vi "ExGraph.vi"() -> ()   [LabVIEW 2018]
uses:
  Lib/STM/Graph/MOKO_Graph_main_STM.ctl
  Lib/STM/Graph/MOKO_Graph_main_ITEM.ctl
  Lib/STM/Grafic/MOKO_Grafic_STM.ctl
  Lib/STM/Grafic/MOKO_Grafic_ITEM.ctl
  Lib/CTL/STM GRAPH.ctl
  Lib/CTL/Graph settings.ctl
  Lib/CTL/Line.ctl
  <vilib>/Utility/miscctls.llb/LVComboBoxStrsAndValuesArrayTypeDef.ctl
  Lib/Windows/Settings/GraphSettings/GraphSettings_STM.ctl
  Lib/Windows/Settings/GraphSettings/GraphSettings_ITEM.ctl
panel:
  in  "Delete":bool
  in  "Screenshot Indicator":bool
  in  "params":string
  in  "STM Graph":T1={"Graph settings"={"Axis X Min"=0.0, "Axis X Name"="", "Axis X Max"=0.0, "Axis Y Min"=0.0, " Axis Y Name"="", "Axis Y Max"=1.0, "Autoscale"=enum."Yes", "Choice Line"=1.0}, "Lines"=[], "Data"=""} {"Lines"."Color" format="%x"}
  out "MOKO_GRAPH_STM":refnum<queue>
  in  "Combo Box":string(combo)
  in  "Base64 String":string
  out "XY Graph":cluster{"Array Ox":dbl[], "Array Oy":dbl[]}[](graph)
  out "String Array Out":string[](array[string])
  in  "NumPlot":dbl
  out "Counter":dbl
  out "Hide/Show Array":dbl[](array[numeric])
  in  "Config":bool
  in  "Start":bool
  out "MOKO_GRAPH_SERVER":refnum<queue>
  in  "Stop":bool
  out "Boolean":bool
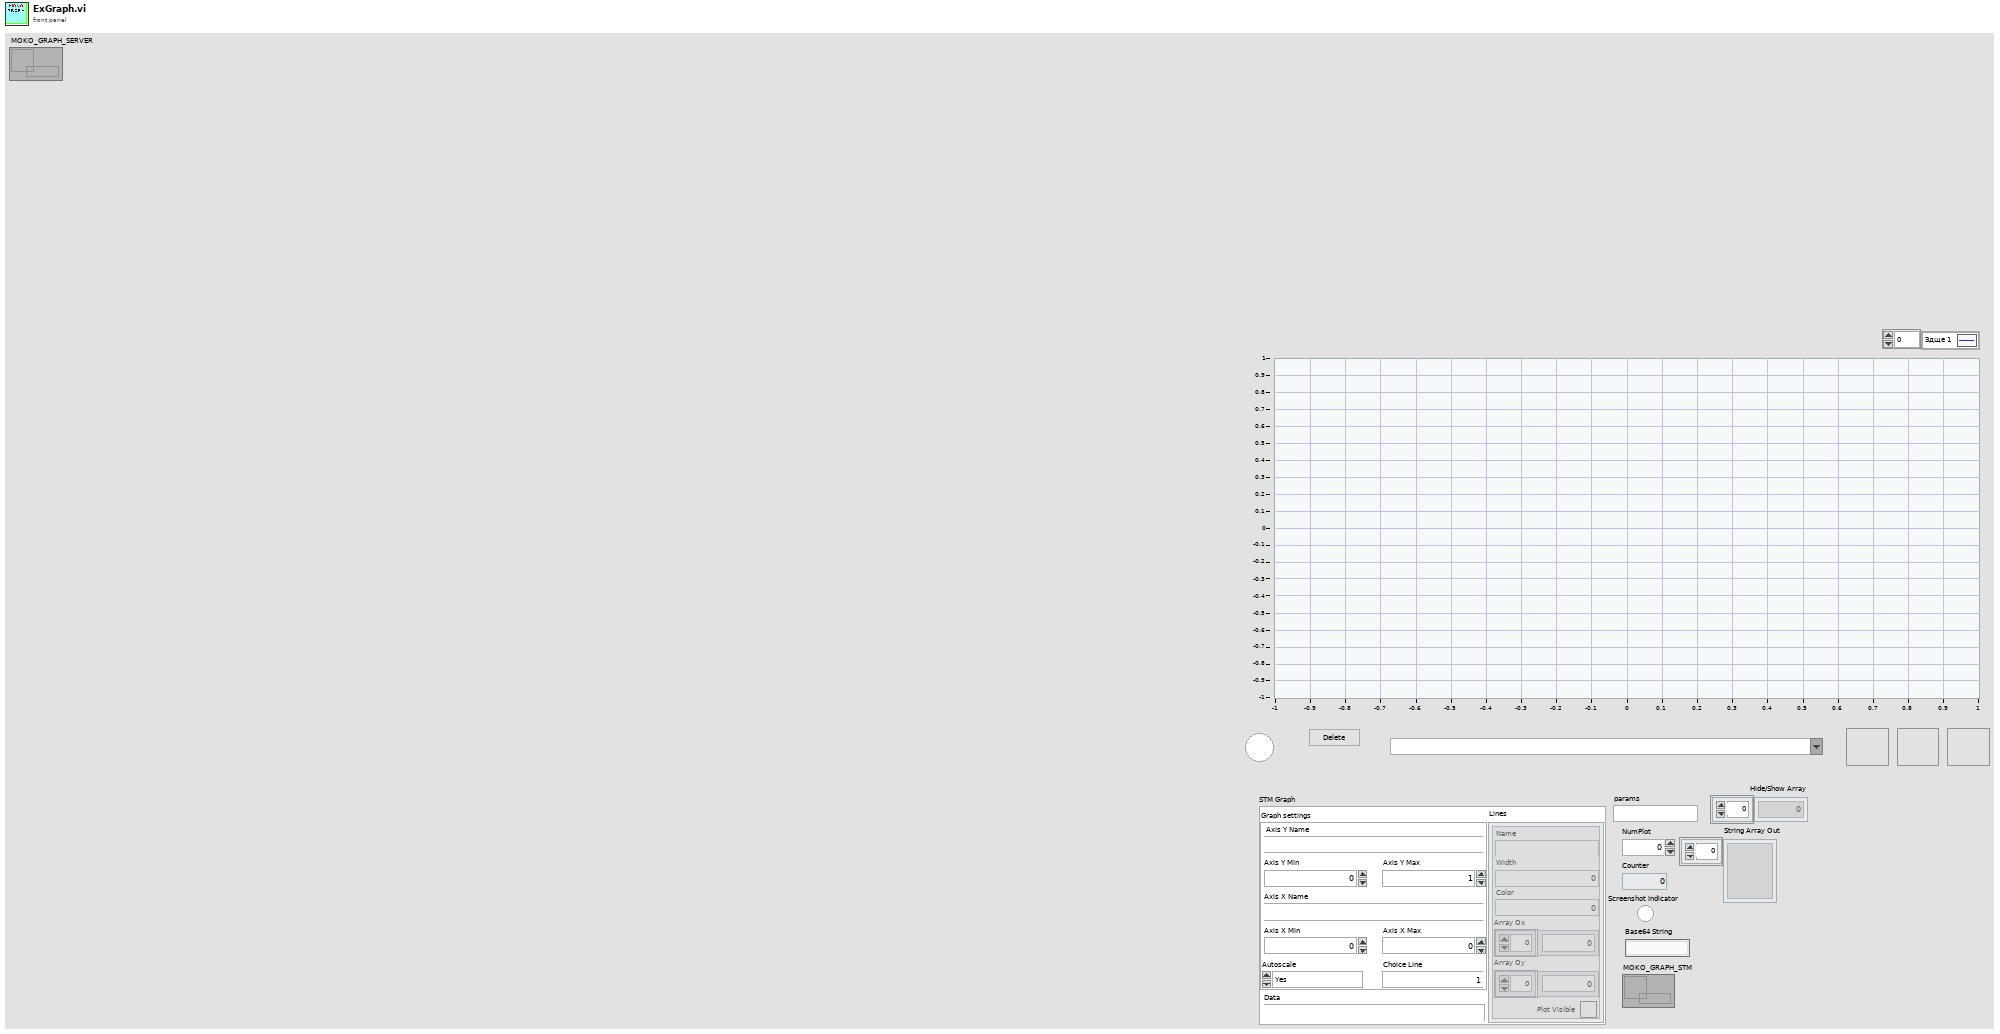
[diagram p1: front panel]
types:
  T1 = typedef "STM GRAPH.ctl" = cluster{"Graph settings":T2, "Lines":T3[], "Data":string}
  T2 = typedef "Graph settings.ctl" = cluster{"Axis X Min":dbl, "Axis X Name":string, "Axis X Max":dbl, "Axis Y Min":dbl, " Axis Y Name":string, "Axis Y Max":dbl, "Autoscale":enum16{"Yes", "No", "Only Oy", "Only Ox"}, "Choice Line":dbl}
  T3 = typedef "Line.ctl" = cluster{"Width":dbl, "Color":i64, "Array Oy":dbl[], "Array Ox":dbl[], "Name":string, "Plot Visible":bool}
  T4 = typedef "MOKO_Grafic_STM.ctl" = cluster{"main stm":T5, "STM Graph":T1}
  T5 = typedef "MOKO_Grafic_ITEM.ctl" = enum16{"idle", "init", "_____ GRAPH STATE_____ ", "Write Graph", "Clear Graph", "close", "Screenshot", "Change Line", "Add Line", "Parse String In", "Add Data", "Change Data", "Graph Settings", "Get Graph Appearance", "Set Graph Appearance", "Delete Data", "Delete Line", "Choose ActPlot", "Set Line Settings", "Increment Smth", "ReWrite Graph", "Autoscale", "Set Autoscale", "Hide Line", "Get Hide Line", "Hide Data", "Show Line", "Get Show Line", "Show Data", "Choose Line", "Change Combo Box", "Send Data", "Receive Data", "Choice Line", "Change Lines"}
  T6 = typedef "MOKO_Graph_main_STM.ctl" = cluster{"main stm":T7, "data":string}
  T7 = typedef "MOKO_Graph_main_ITEM.ctl" = enum16{"idle", "Graph read", "Graph write"}
  T8 = typedef "LVComboBoxStrsAndValuesArrayTypeDef.ctl" = cluster{"String":string, "Value":string}[]
  T9 = typedef "GraphSettings_STM.ctl" = cluster{"main stm":T10, "STM Graph":T1}
  T10 = typedef "GraphSettings_ITEM.ctl" = enum16{"idle", "init", "close", "_____ GRAPH STATE_____ ", "Receive Data", "Send Data", "Change Line", "Delete Line", "Add Line", "Find Max", "Change Color", "Choice Line"}
  T11 = typedef "imagedata.ctl" = cluster{"image type":i32, "image depth":i32, "image":u8[], "mask":u8[], "colors":u32[], "Rectangle":cluster{"left":i16, "top":i16, "right":i16, "bottom":i16}}
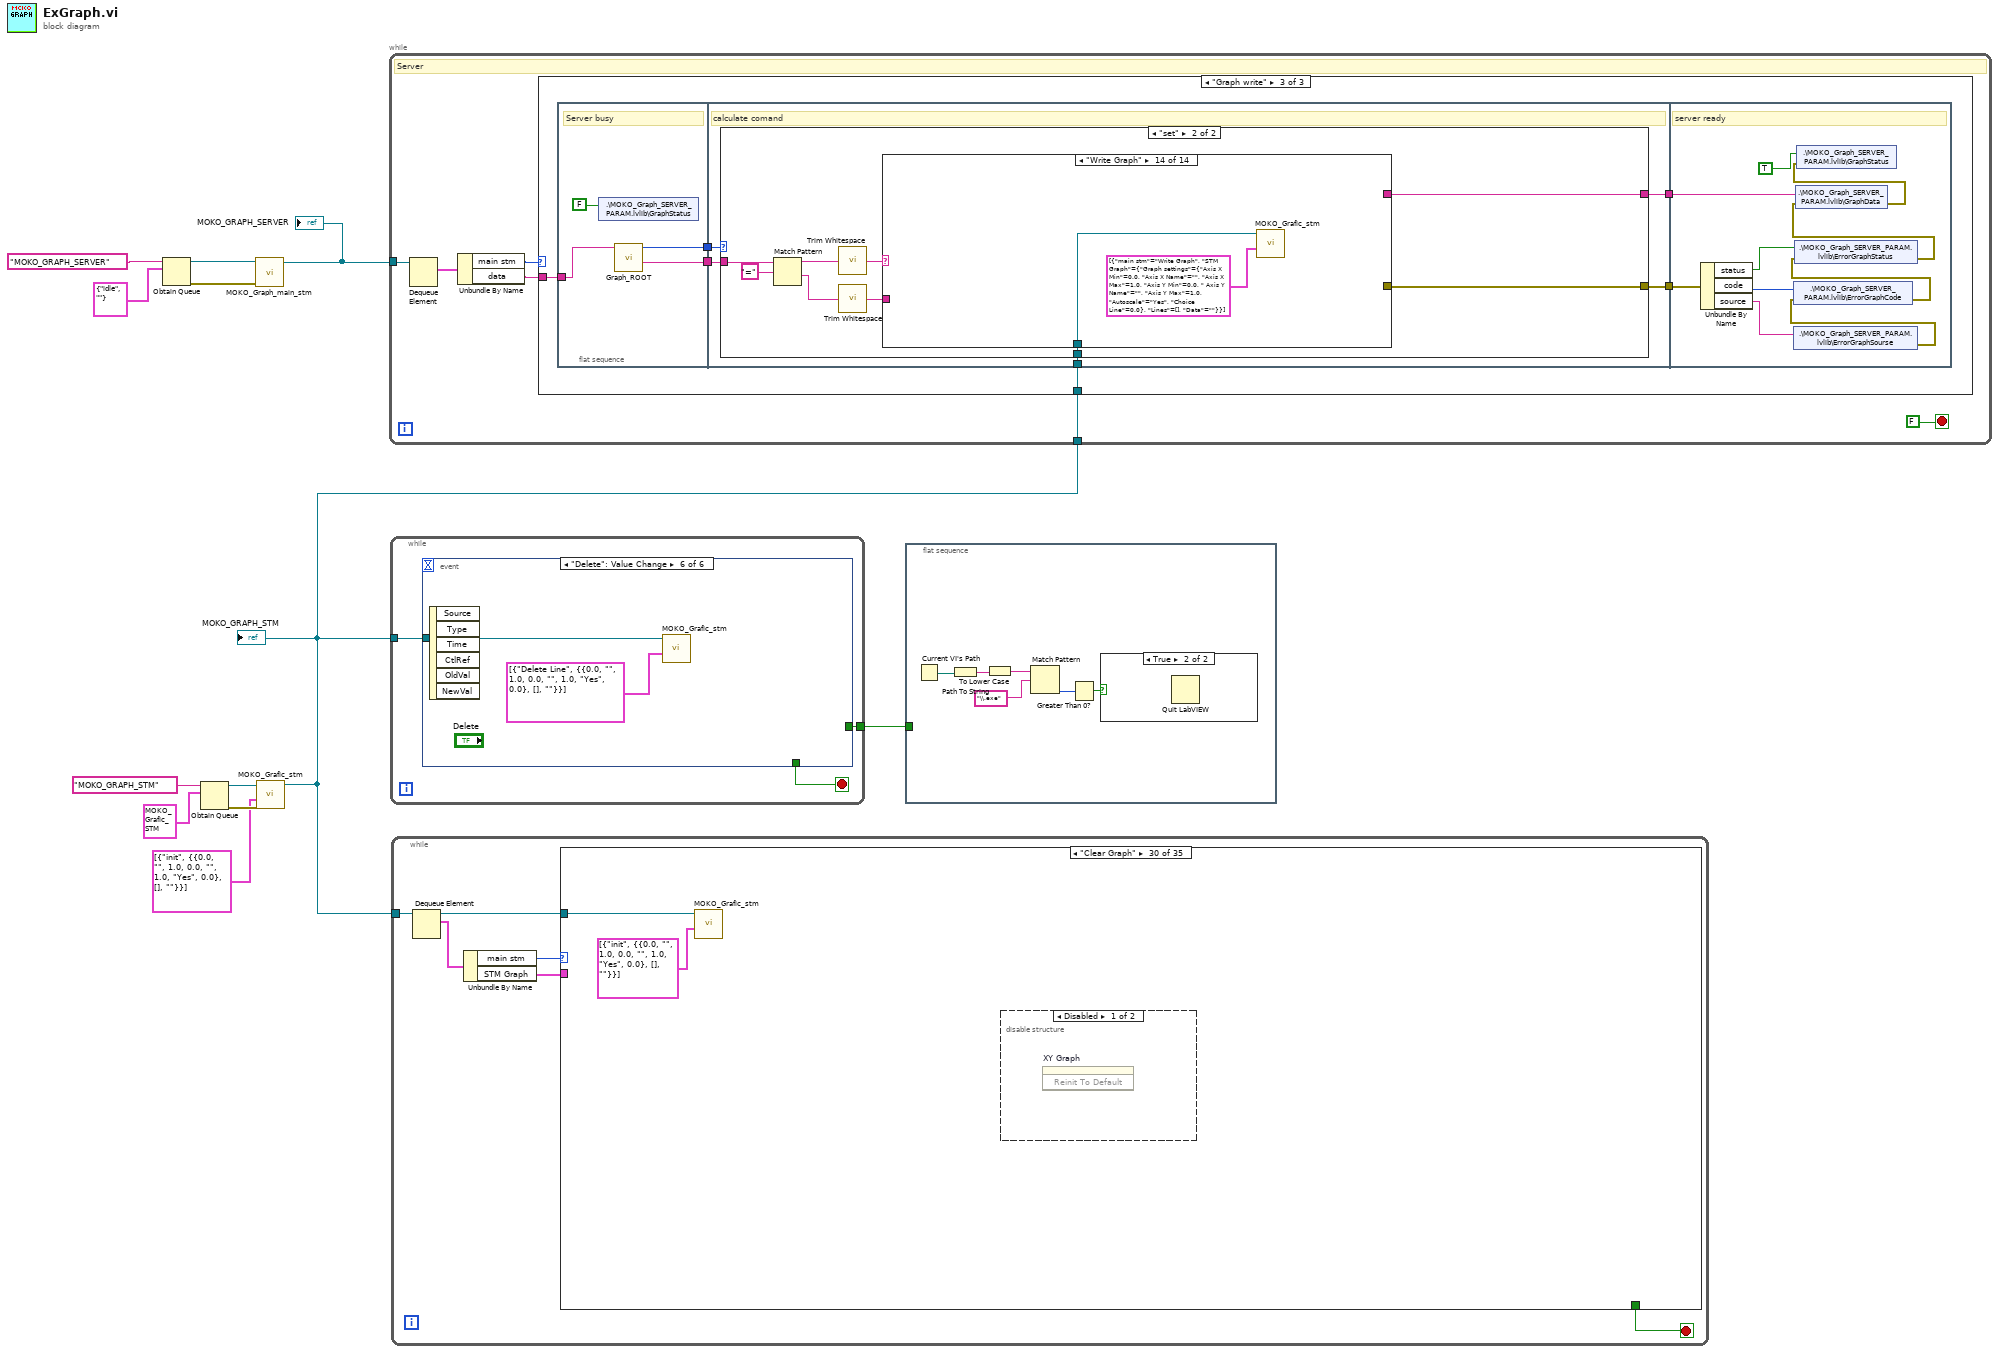
[diagram p0: block diagram]
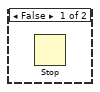
[diagram p2: hidden frame]
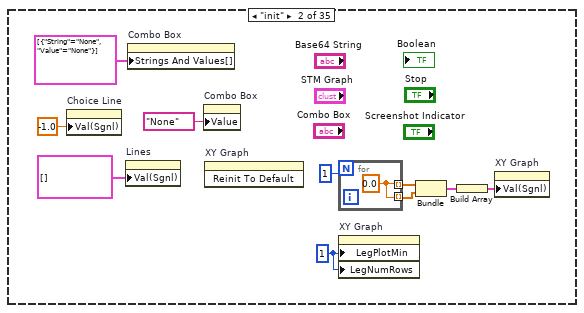
[diagram p4: hidden frame]
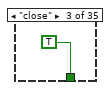
[diagram p5: hidden frame]
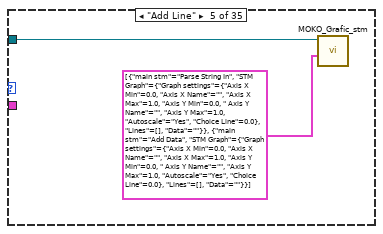
[diagram p7: hidden frame]
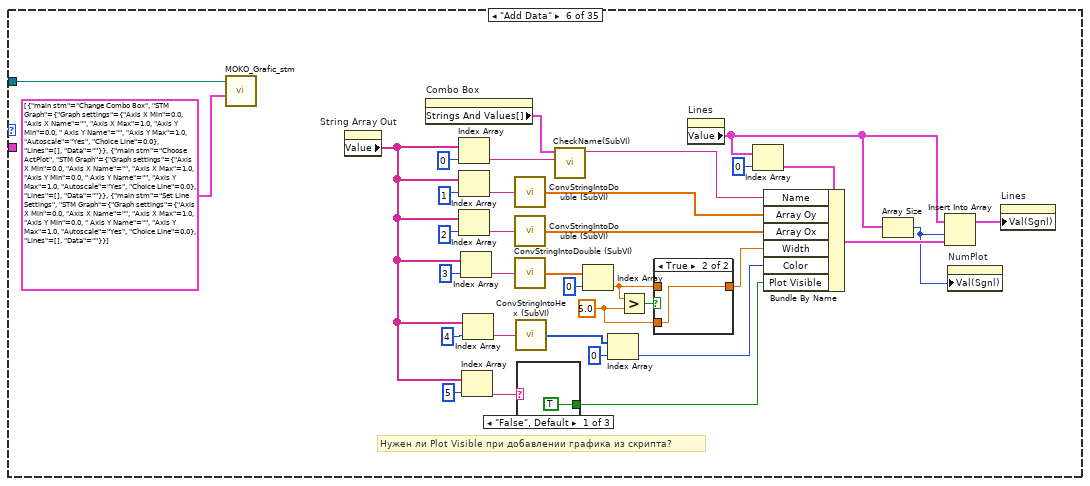
[diagram p8: hidden frame]
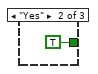
[diagram p10: hidden frame]
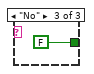
[diagram p11: hidden frame]
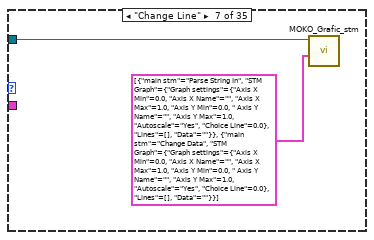
[diagram p12: hidden frame]
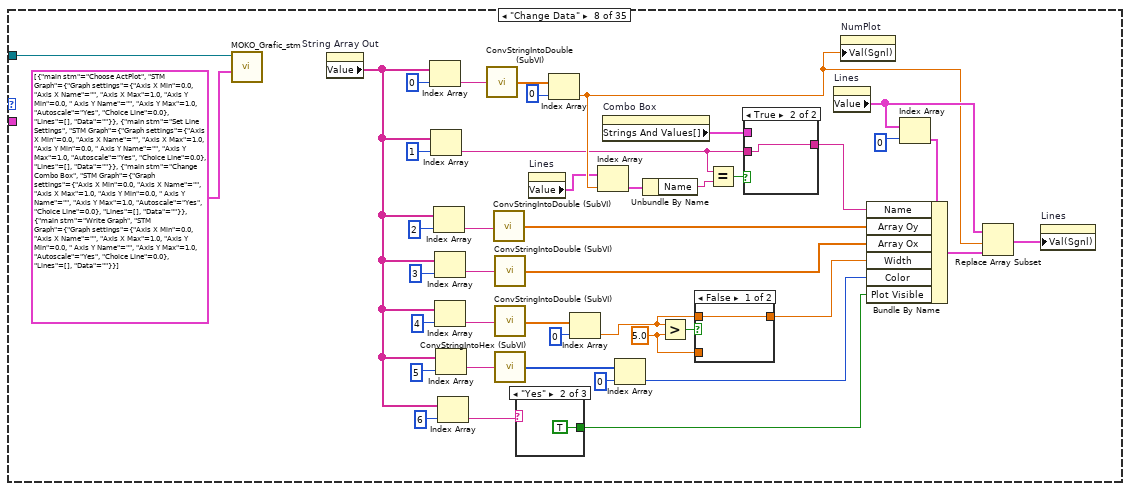
[diagram p13: hidden frame]
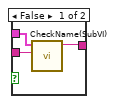
[diagram p15: hidden frame]
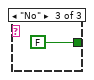
[diagram p17: hidden frame]
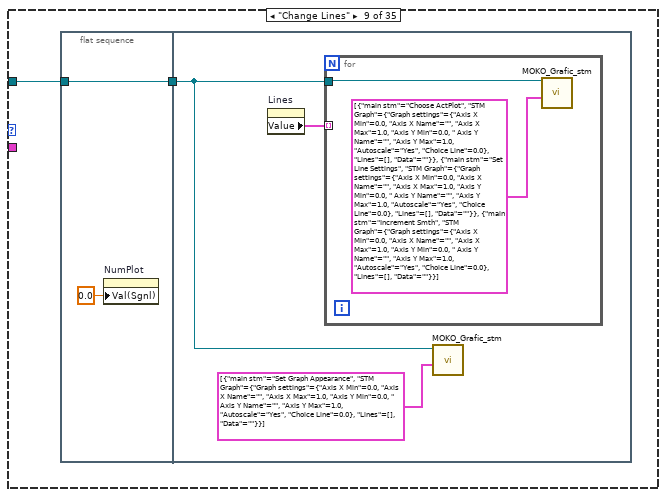
[diagram p18: hidden frame]
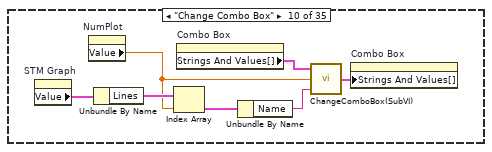
[diagram p19: hidden frame]
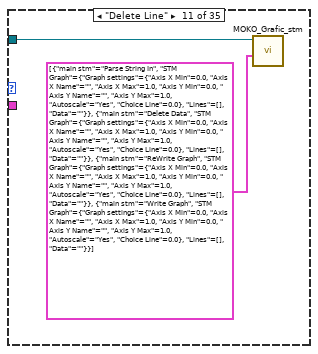
[diagram p20: hidden frame]
diagram:
  n1 = Obtain Queue(name (unnamed)="MOKO_GRAPH_SERVER", element data type=T6 {"main stm"=enum."idle", "data"=""} ("MOKO_SE_STM")) -> (queue out=w10:refnum<queue>, error out=w9:errorcluster)  [unwired: 3 in, 1 out]
  n2 = Obtain Queue(name (unnamed)="MOKO_GRAPH_STM", element data type=T4 {"main stm"=enum."idle", "STM Graph"={"Graph settings"={"Axis X Min"=0.0, "Axis X Name"="", "Axis X Max"=1.0, "Axis Y Min"=0.0, " Axis Y Name"="", "Axis Y Max"=1.0, "Autoscale"=enum."Yes", "Choice Line"=0.0}, "Lines"=[], "Data"=""}} ("MOKO_SE_STM")) -> (queue out=w7:refnum<queue>, error out=w6:errorcluster)  [unwired: 3 in, 1 out]
  n3 = call "MOKO_Graph_main_stm.vi"("error in"=w9, "queue in"=w10) -> ("queue out"=w4:refnum<queue>)  [unwired: 8 in, 1 out]
  "MOKO_GRAPH_SERVER" <- w4
  n4 = call "MOKO_Grafic_stm.vi"("error in"=w6, "StateMachineSteps"=T4[] [{"main stm"=enum."init", "STM Graph"={"Graph settings"={"Axis X Min"=0.0, "Axis X Name"="", "Axis X Max"=1.0, "Axis Y Min"=0.0, " Axis Y Name"="", "Axis Y Max"=1.0, "Autoscale"=enum."Yes", "Choice Line"=0.0}, "Lines"=[], "Data"=""}}], "queue in"=w7) -> ("queue out"=w1:refnum<queue>)  [unwired: 7 in, 1 out]
  "MOKO_GRAPH_STM" <- w1
  n5 = while {
    tunnel: w4 -> [w17]
    tunnel: w1 -> [w13]
    stop <- FALSE stop-if-true
    # "Server"
    n6 = Dequeue Element(queue=w17) -> (element=w18:T6)  [unwired: 2 in, 3 out]
    n7 = Unbundle By Name(w18) -> ("main stm"=w16:T7, "data"=w15:string)
    n8 = case shown="\"Graph write\"" w16 {
      tunnel: w15 -> [_ _ w22]
      tunnel: w13 -> [_ _ w19]
      frame "idle", Default {
      }
      frame "Graph read" {
      }
      frame "Graph write" {
        n9 = flat-sequence {
          tunnel: w22 -> [w27]
          tunnel: [w26] -> w21
          tunnel: [w25] -> w20
          tunnel: [w30] -> w24
          tunnel: [w33] -> w23
          tunnel: w21 -> [w32]
          tunnel: w20 -> [w31]
          tunnel: w19 -> [w29]
          tunnel: w24 -> [w107]
          tunnel: w23 -> [w111]
          frame #0 {
            # "Server busy"
            n10 = shared-variable ".\\MOKO_Graph_SERVER_PARAM.lvlib\\GraphStatus"(FALSE) -> ()  [unwired: 1 in, 1 out]
            n11 = call "Graph_ROOT.vi"("data"=w27) -> ("command"=w25:string, "Mode out"=w26:enum16{"get", "set", "close", "Init", "Check"})  [unwired: 7 in, 2 out]
          }
          frame #1 {
            # "calculate comand"
            n12 = case shown="\"set\"" w32 {
              tunnel: [_ w61] -> w33
              tunnel: w31 -> [w37 w59]
              tunnel: [w41 w54] -> w30
              tunnel: w29 -> [w34 w53]
              frame "get", Default {
                n13 = Match Pattern(string=w37, regular expression="=") -> (before substring=w38:string, after substring=w40:string)  [unwired: 1 in, 2 out]
                n14 = call <vilib>:"Trim Whitespace.vi"("string"=w38) -> ("trimmed string"=w36:string)  [unwired: 1 in]
                n15 = call <vilib>:"Trim Whitespace.vi"("string"=w40) -> ("trimmed string"=w35:string)  [unwired: 1 in]
                n16 = case shown="\"InstantScreenshot\"" w36 {
                  tunnel: [_ w43 _] -> w41
                  tunnel: w35 -> [_ _ w50]
                  tunnel: w34 -> [_ w42 _]
                  frame "False", Default {
                  }
                  frame "InstantScreenshot" {
                    n17 = flat-sequence {
                      tunnel: w42 -> [w45]
                      tunnel: [w49] -> w43
                      frame #0 {
                        n18 = property on="Screenshot Indicator" class="Bool (strict)"("Val(Sgnl)"=TRUE ("Value (Signaling)")) -> ()  [unwired: 2 in, 2 out]
                        n19 = call "MOKO_Grafic_stm.vi"("StateMachineSteps"=T4[] [{"main stm"=enum."Screenshot", "STM Graph"={"Graph settings"={"Axis X Min"=0.0, "Axis X Name"="", "Axis X Max"=1.0, "Axis Y Min"=0.0, " Axis Y Name"="", "Axis Y Max"=1.0, "Autoscale"=enum."Yes", "Choice Line"=0.0}, "Lines"=[], "Data"=""}}], "queue in"=w45) -> ()  [unwired: 8 in, 2 out]
                      }
                      frame #1 {
                        n20 = while {
                          stop <- w47 stop-if-true
                          n21 = property on="Screenshot Indicator" class="Bool (strict)"() -> ("Value"=w48:bool)  [unwired: 2 in, 2 out]
                          n22 = Not(x=w48) -> (.not. x?=w47:bool)
                        }
                      }
                      frame #2 {
                        n23 = property on="Base64 String" class="Str"() -> ("Value"=w49:string)  [unwired: 2 in, 2 out]
                      }
                    }
                  }
                  frame "Max" {
                    n24 = flat-sequence {
                      tunnel: w50 -> [w51]
                      frame #0 {
                        n25 = property on="params" class="Str"("Val(Sgnl)"=w51) -> ()  [unwired: 2 in, 2 out]
                      }
                      frame #1 {
                      }
                      frame #2 {
                        n26 = while {
                          stop <- FALSE stop-if-true
                        }
                      }
                      frame #3 {
                      }
                    }
                  }
                }
              }
              frame "set" {
                n27 = Match Pattern(string=w59, regular expression="=") -> (before substring=w57:string, after substring=w60:string)  [unwired: 1 in, 2 out]
                n28 = call <vilib>:"Trim Whitespace.vi"("string"=w57) -> ("trimmed string"=w56:string)  [unwired: 1 in]
                n29 = call <vilib>:"Trim Whitespace.vi"("string"=w60) -> ("trimmed string"=w55:string)  [unwired: 1 in]
                n30 = case shown="\"Write Graph\"" w56 {
                  tunnel: [_ errorcluster {"status"=FALSE, "code"=0, "source"=""} ("error out") _ _ _ _ _ _ _ _ _ _ _ _] -> w61
                  tunnel: w55 -> [_ _ w65 w70 _ w77 w82 w87 _ w94 w99 w103 _ _]
                  tunnel: [_ "" _ _ _ _ _ _ _ _ _ _ _ _] -> w54
                  tunnel: w53 -> [_ _ w64 w69 w74 w76 w81 w86 w91 w93 w98 _ _ w105]
                  frame "False", Default {
                  }
                  frame "ChangeLedLoop" {
                  }
                  frame "Autoscale" {
                    n31 = flat-sequence {
                      tunnel: w65 -> [w66]
                      tunnel: w64 -> [w67]
                      frame #0 {
                        n32 = property on="params" class="Str"("Val(Sgnl)"=w66) -> ()  [unwired: 2 in, 2 out]
                      }
                      frame #1 {
                        n33 = call "MOKO_Grafic_stm.vi"("StateMachineSteps"=T4[] [{"main stm"=enum."Autoscale", "STM Graph"={"Graph settings"={"Axis X Min"=0.0, "Axis X Name"="", "Axis X Max"=1.0, "Axis Y Min"=0.0, " Axis Y Name"="", "Axis Y Max"=1.0, "Autoscale"=enum."Yes", "Choice Line"=0.0}, "Lines"=[], "Data"=""}}], "queue in"=w67) -> ()  [unwired: 8 in, 2 out]
                      }
                    }
                  }
                  frame "Add Line" {
                    n34 = flat-sequence {
                      tunnel: w70 -> [w71]
                      tunnel: w69 -> [w72]
                      frame #0 {
                        n35 = property on="params" class="Str"("Val(Sgnl)"=w71) -> ()  [unwired: 2 in, 2 out]
                      }
                      frame #1 {
                        n36 = call "MOKO_Grafic_stm.vi"("StateMachineSteps"=T4[] [{"main stm"=enum."Add Line", "STM Graph"={"Graph settings"={"Axis X Min"=0.0, "Axis X Name"="", "Axis X Max"=1.0, "Axis Y Min"=0.0, " Axis Y Name"="", "Axis Y Max"=1.0, "Autoscale"=enum."Yes", "Choice Line"=0.0}, "Lines"=[], "Data"=""}}], "queue in"=w72) -> ()  [unwired: 8 in, 2 out]
                      }
                    }
                  }
                  frame "Screenshot" {
                    n37 = call "MOKO_Grafic_stm.vi"("StateMachineSteps"=T4[] [{"main stm"=enum."Screenshot", "STM Graph"={"Graph settings"={"Axis X Min"=0.0, "Axis X Name"="", "Axis X Max"=1.0, "Axis Y Min"=0.0, " Axis Y Name"="", "Axis Y Max"=1.0, "Autoscale"=enum."Yes", "Choice Line"=0.0}, "Lines"=[], "Data"=""}}], "queue in"=w74) -> ()  [unwired: 8 in, 2 out]
                  }
                  frame "Change Line" {
                    n38 = flat-sequence {
                      tunnel: w77 -> [w78]
                      tunnel: w76 -> [w79]
                      tunnel: [w79] -> _
                      frame #0 {
                        n39 = property on="params" class="Str"("Val(Sgnl)"=w78) -> ()  [unwired: 2 in, 2 out]
                      }
                      frame #1 {
                        n40 = call "MOKO_Grafic_stm.vi"("StateMachineSteps"=T4[] [{"main stm"=enum."Change Line", "STM Graph"={"Graph settings"={"Axis X Min"=0.0, "Axis X Name"="", "Axis X Max"=1.0, "Axis Y Min"=0.0, " Axis Y Name"="", "Axis Y Max"=1.0, "Autoscale"=enum."Yes", "Choice Line"=0.0}, "Lines"=[], "Data"=""}}], "queue in"=w79) -> ()  [unwired: 8 in, 2 out]
                      }
                    }
                  }
                  frame "Add Graph Settings" {
                    n41 = flat-sequence {
                      tunnel: w82 -> [w83]
                      tunnel: w81 -> [w84]
                      frame #0 {
                        n42 = property on="params" class="Str"("Val(Sgnl)"=w83) -> ()  [unwired: 2 in, 2 out]
                      }
                      frame #1 {
                        n43 = call "MOKO_Grafic_stm.vi"("StateMachineSteps"=T4[] [{"main stm"=enum."Graph Settings", "STM Graph"={"Graph settings"={"Axis X Min"=0.0, "Axis X Name"="", "Axis X Max"=1.0, "Axis Y Min"=0.0, " Axis Y Name"="", "Axis Y Max"=1.0, "Autoscale"=enum."Yes", "Choice Line"=0.0}, "Lines"=[], "Data"=""}}], "queue in"=w84) -> ()  [unwired: 8 in, 2 out]
                      }
                    }
                  }
                  frame "Delete Line" {
                    n44 = flat-sequence {
                      tunnel: w87 -> [w88]
                      tunnel: w86 -> [w89]
                      frame #0 {
                        n45 = property on="params" class="Str"("Val(Sgnl)"=w88) -> ()  [unwired: 2 in, 2 out]
                      }
                      frame #1 {
                        n46 = call "MOKO_Grafic_stm.vi"("StateMachineSteps"=T4[] [{"main stm"=enum."Delete Line", "STM Graph"={"Graph settings"={"Axis X Min"=0.0, "Axis X Name"="", "Axis X Max"=1.0, "Axis Y Min"=0.0, " Axis Y Name"="", "Axis Y Max"=1.0, "Autoscale"=enum."Yes", "Choice Line"=0.0}, "Lines"=[], "Data"=""}}], "queue in"=w89) -> ()  [unwired: 8 in, 2 out]
                      }
                    }
                  }
                  frame "Clear Graph" {
                    n47 = call "MOKO_Grafic_stm.vi"("StateMachineSteps"=T4[] [{"main stm"=enum."Clear Graph", "STM Graph"={"Graph settings"={"Axis X Min"=0.0, "Axis X Name"="", "Axis X Max"=1.0, "Axis Y Min"=0.0, " Axis Y Name"="", "Axis Y Max"=1.0, "Autoscale"=enum."Yes", "Choice Line"=0.0}, "Lines"=[], "Data"=""}}], "queue in"=w91) -> ()  [unwired: 8 in, 2 out]
                  }
                  frame "Hide Line" {
                    n48 = flat-sequence {
                      tunnel: w94 -> [w95]
                      tunnel: w93 -> [w96]
                      frame #0 {
                        n49 = property on="params" class="Str"("Val(Sgnl)"=w95) -> ()  [unwired: 2 in, 2 out]
                      }
                      frame #1 {
                        n50 = call "MOKO_Grafic_stm.vi"("StateMachineSteps"=T4[] [{"main stm"=enum."Hide Line", "STM Graph"={"Graph settings"={"Axis X Min"=0.0, "Axis X Name"="", "Axis X Max"=1.0, "Axis Y Min"=0.0, " Axis Y Name"="", "Axis Y Max"=1.0, "Autoscale"=enum."Yes", "Choice Line"=0.0}, "Lines"=[], "Data"=""}}], "queue in"=w96) -> ()  [unwired: 8 in, 2 out]
                      }
                    }
                  }
                  frame "Show Line" {
                    n51 = flat-sequence {
                      tunnel: w99 -> [w100]
                      tunnel: w98 -> [w101]
                      frame #0 {
                        n52 = property on="params" class="Str"("Val(Sgnl)"=w100) -> ()  [unwired: 2 in, 2 out]
                      }
                      frame #1 {
                        n53 = call "MOKO_Grafic_stm.vi"("StateMachineSteps"=T4[] [{"main stm"=enum."Show Line", "STM Graph"={"Graph settings"={"Axis X Min"=0.0, "Axis X Name"="", "Axis X Max"=1.0, "Axis Y Min"=0.0, " Axis Y Name"="", "Axis Y Max"=1.0, "Autoscale"=enum."Yes", "Choice Line"=0.0}, "Lines"=[], "Data"=""}}], "queue in"=w101) -> ()  [unwired: 8 in, 2 out]
                      }
                    }
                  }
                  frame "Max" {
                    n54 = flat-sequence {
                      tunnel: w103 -> [w104]
                      frame #0 {
                        n55 = property on="params" class="Str"("Val(Sgnl)"=w104) -> ()  [unwired: 2 in, 2 out]
                      }
                      frame #1 {
                      }
                    }
                  }
                  frame "Stop Graph" {
                  }
                  frame "Write Graph" {
                    n56 = call "MOKO_Grafic_stm.vi"("StateMachineSteps"=T4[] [{"main stm"=enum."Write Graph", "STM Graph"={"Graph settings"={"Axis X Min"=0.0, "Axis X Name"="", "Axis X Max"=1.0, "Axis Y Min"=0.0, " Axis Y Name"="", "Axis Y Max"=1.0, "Autoscale"=enum."Yes", "Choice Line"=0.0}, "Lines"=[], "Data"=""}}], "queue in"=w105) -> ()  [unwired: 8 in, 2 out]
                  }
                }
              }
            }
          }
          frame #2 {
            # "server ready"
            n57 = Unbundle By Name(w111) -> ("status"=w110:bool, "code"=w109:i32, "source"=w108:string)
            n58 = shared-variable ".\\MOKO_Graph_SERVER_PARAM.lvlib\\ErrorGraphSourse"(w108) -> (error out=w113:errorcluster)  [unwired: 1 in]
            n59 = shared-variable ".\\MOKO_Graph_SERVER_PARAM.lvlib\\ErrorGraphCode"(w109, error in=w113) -> (error out=w114:errorcluster)
            n60 = shared-variable ".\\MOKO_Graph_SERVER_PARAM.lvlib\\ErrorGraphStatus"(w110, error in=w114) -> (error out=w115:errorcluster)
            n61 = shared-variable ".\\MOKO_Graph_SERVER_PARAM.lvlib\\GraphData"(w107, error in=w115) -> (error out=w116:errorcluster)
            n62 = shared-variable ".\\MOKO_Graph_SERVER_PARAM.lvlib\\GraphStatus"(TRUE, error in=w116) -> ()  [unwired: 1 out]
          }
        }
      }
    }
  }
  n63 = while {
    tunnel: [w118] -> w5
    tunnel: w1 -> [w117]
    stop <- w119 stop-if-true
    n64 = event shown="[5] \"Delete\": Value Change" {
      selector: _ -> [_ _ _ _ _ _]
      dyn-events: _ -> [_ _ _ _ _ _]
      timeout: _ -> [_ _ _ _ _ _]
      tunnel: [_ _ _ w125 _ _] -> w119
      tunnel: [_ _ _ w125 _ _] -> w118
      tunnel: w117 -> [_ w120 w122 w124 w130 w132]
      event Timeout {
        n65 = event-data() -> ()  [unwired: 1 in, 3 out]
      }
      event "Start": Value Change {
        n66 = event-data() -> ()  [unwired: 1 in, 6 out]
        n67 = call "MOKO_Grafic_stm.vi"("StateMachineSteps"=T4[] [{"main stm"=enum."Write Graph", "STM Graph"={"Graph settings"={"Axis X Min"=0.0, "Axis X Name"="", "Axis X Max"=1.0, "Axis Y Min"=0.0, " Axis Y Name"="", "Axis Y Max"=1.0, "Autoscale"=enum."Yes", "Choice Line"=0.0}, "Lines"=[], "Data"=""}}], "queue in"=w120) -> ()  [unwired: 8 in, 2 out]
      }
      event "Combo Box": Value Change {
        n68 = event-data() -> ()  [unwired: 1 in, 6 out]
        n69 = call "MOKO_Grafic_stm.vi"("StateMachineSteps"=T4[] [{"main stm"=enum."Choice Line", "STM Graph"={"Graph settings"={"Axis X Min"=0.0, "Axis X Name"="", "Axis X Max"=1.0, "Axis Y Min"=0.0, " Axis Y Name"="", "Axis Y Max"=1.0, "Autoscale"=enum."Yes", "Choice Line"=0.0}, "Lines"=[], "Data"=""}}], "queue in"=w122) -> ()  [unwired: 8 in, 2 out]
      }
      event Panel Close? {
        w125 = TRUE
        n70 = event-data() -> ()  [unwired: 1 in, 4 out]
        n71 = call "MOKO_Grafic_stm.vi"("StateMachineSteps"=T4[] [{"main stm"=enum."close", "STM Graph"={"Graph settings"={"Axis X Min"=0.0, "Axis X Name"="", "Axis X Max"=1.0, "Axis Y Min"=0.0, " Axis Y Name"="", "Axis Y Max"=1.0, "Autoscale"=enum."Yes", "Choice Line"=0.0}, "Lines"=[], "Data"=""}}], "FNs"=enum16{"Back", "Front", "Replace"}."Replace", "queue in"=w124) -> ()  [unwired: 7 in, 2 out]
        n72 = event-data("Discard?"=FALSE) -> ()  [unwired: 1 in, 1 out]
      }
      event "Config": Value Change {
        n73 = event-data() -> ()  [unwired: 1 in, 6 out]
        n74 = call "MOKO_Grafic_stm.vi"("StateMachineSteps"=T4[] [{"main stm"=enum."Send Data", "STM Graph"={"Graph settings"={"Axis X Min"=0.0, "Axis X Name"="", "Axis X Max"=1.0, "Axis Y Min"=0.0, " Axis Y Name"="", "Axis Y Max"=1.0, "Autoscale"=enum."Yes", "Choice Line"=0.0}, "Lines"=[], "Data"=""}}], "queue in"=w130) -> ()  [unwired: 8 in, 2 out]
      }
      event "Delete": Value Change {
        n75 = event-data() -> ()  [unwired: 1 in, 6 out]
        n76 = call "MOKO_Grafic_stm.vi"("StateMachineSteps"=T4[] [{"main stm"=enum."Delete Line", "STM Graph"={"Graph settings"={"Axis X Min"=0.0, "Axis X Name"="", "Axis X Max"=1.0, "Axis Y Min"=0.0, " Axis Y Name"="", "Axis Y Max"=1.0, "Autoscale"=enum."Yes", "Choice Line"=0.0}, "Lines"=[], "Data"=""}}], "queue in"=w132) -> ()  [unwired: 8 in, 2 out]
      }
    }
  }
  n77 = while {
    tunnel: w1 -> [w138]
    stop <- w133 stop-if-true
    n78 = Dequeue Element(queue=w138) -> (queue out=w134:refnum<queue>, element=w137:T4)  [unwired: 2 in, 2 out]
    n79 = Unbundle By Name(w137) -> ("main stm"=w136:T5, "STM Graph"=w135:T1)
    n80 = case shown="\"Clear Graph\"" w136 {
      tunnel: w134 -> [_ _ _ _ w152 w187 w194 w237 w247 _ w263 _ _ _ _ _ w379 w396 w433 _ w435 _ _ _ _ _ w455 _ w463 w469 _ w477 _ w497 _]
      tunnel: w135 -> [_ _ _ _ _ _ _ _ _ _ _ _ _ _ _ _ _ _ _ _ _ _ _ _ _ _ _ _ _ _ _ w478 _ _ _]
      tunnel: [_ _ TRUE _ _ _ _ _ _ _ _ _ _ _ _ _ _ _ _ _ _ _ _ _ _ _ _ _ _ _ _ _ _ _ _] -> w133
      frame "idle", Default {
      }
      frame "init" {
        w142 = u32 1 ("Legend:Plot Minimum")
        n81 = property on="Choice Line" class="DigNum (strict)"("Val(Sgnl)"=-1.0 ("Value (Signaling)")) -> ()  [unwired: 2 in, 2 out]
        n82 = property on="Lines" class="Arr (strict)"("Val(Sgnl)"=T3[] [] ("Value (Signaling)")) -> ()  [unwired: 2 in, 2 out]
        n83 = property on="Combo Box" class="CmbBox"("Strings And Values[]"=T8 [{"String"="None", "Value"="None"}] ("Strings And Values []")) -> ()  [unwired: 2 in, 2 out]
        n84 = property on="Combo Box" class="CmbBox"("Value"="None" ("Combo Box")) -> ()  [unwired: 2 in, 2 out]
        n85 = invoke on="XY Graph" class="XYGraph (strict)" method="Reinit To Default"() -> ()  [unwired: 3 in, 3 out]
        n86 = for {
          N: 1 -> [_]
          tunnel: [w149] -> w145 mode=indexing
          tunnel: [w149] -> w144 mode=indexing
          w149 = 0.0 ("number: 0 to 1")
        }
        n87 = property on="XY Graph" class="XYGraph (strict)"("LegPlotMin"=w142, "LegNumRows"=w142) -> ()  [unwired: 2 in, 2 out]
        n88 = Bundle(w145, w144) -> (w141:cluster{dbl[], dbl[]})  [unwired: 1 in]
        n89 = Build Array(w141) -> (w140:cluster{dbl[], dbl[]}[])
        n90 = property on="XY Graph" class="XYGraph (strict)"("Val(Sgnl)"=w140) -> ()  [unwired: 2 in, 2 out]
      }
      frame "close" {
      }
      frame "_____ GRAPH STATE_____ " {
      }
      frame "Add Line" {
        n91 = call "MOKO_Grafic_stm.vi"("StateMachineSteps"=T4[] [{"main stm"=enum."Parse String In", "STM Graph"={"Graph settings"={"Axis X Min"=0.0, "Axis X Name"="", "Axis X Max"=1.0, "Axis Y Min"=0.0, " Axis Y Name"="", "Axis Y Max"=1.0, "Autoscale"=enum."Yes", "Choice Line"=0.0}, "Lines"=[], "Data"=""}}, {"main stm"=enum."Add Data", "STM Graph"={"Graph settings"={"Axis X Min"=0.0, "Axis X Name"="", "Axis X Max"=1.0, "Axis Y Min"=0.0, " Axis Y Name"="", "Axis Y Max"=1.0, "Autoscale"=enum."Yes", "Choice Line"=0.0}, "Lines"=[], "Data"=""}}], "queue in"=w152) -> ()  [unwired: 8 in, 2 out]
      }
      frame "Add Data" {
        w161 = 5.0 ("y")
        # "Нужен ли Plot Visible при добавлении графика из скрипта?"
        n92 = call "MOKO_Grafic_stm.vi"("StateMachineSteps"=T4[] [{"main stm"=enum."Change Combo Box", "STM Graph"={"Graph settings"={"Axis X Min"=0.0, "Axis X Name"="", "Axis X Max"=1.0, "Axis Y Min"=0.0, " Axis Y Name"="", "Axis Y Max"=1.0, "Autoscale"=enum."Yes", "Choice Line"=0.0}, "Lines"=[], "Data"=""}}, {"main stm"=enum."Choose ActPlot", "STM Graph"={"Graph settings"={"Axis X Min"=0.0, "Axis X Name"="", "Axis X Max"=1.0, "Axis Y Min"=0.0, " Axis Y Name"="", "Axis Y Max"=1.0, "Autoscale"=enum."Yes", "Choice Line"=0.0}, "Lines"=[], "Data"=""}}, {"main stm"=enum."Set Line Settings", "STM Graph"={"Graph settings"={"Axis X Min"=0.0, "Axis X Name"="", "Axis X Max"=1.0, "Axis Y Min"=0.0, " Axis Y Name"="", "Axis Y Max"=1.0, "Autoscale"=enum."Yes", "Choice Line"=0.0}, "Lines"=[], "Data"=""}}], "queue in"=w187) -> ()  [unwired: 8 in, 2 out]
        n93 = property on="String Array Out" class="Arr (strict)"() -> ("Value"=w156:string[])  [unwired: 2 in, 2 out]
        n94 = property on="Combo Box" class="CmbBox"() -> ("Strings And Values[]"=w165:T8)  [unwired: 2 in, 2 out]
        n95 = Index Array(array=w156, index=0) -> (element=w167:string)
        n96 = Index Array(array=w156, index=1) -> (element=w181:string)
        n97 = Index Array(array=w156, index=2) -> (element=w179:string)
        n98 = Index Array(array=w156, index=3) -> (element=w172:string)
        n99 = Index Array(array=w156, index=5) -> (element=w169:string)
        n100 = Index Array(array=w156, index=4) -> (element=w157:string)
        n101 = call "ConvStringIntoDouble (SubVI).vi"("String In"=w181) -> ("Array Out"=w180:dbl[])
        n102 = call "ConvStringIntoDouble (SubVI).vi"("String In"=w179) -> ("Array Out"=w178:dbl[])
        n103 = call "ConvStringIntoDouble (SubVI).vi"("String In"=w172) -> ("Array Out"=w171:dbl[])
        n104 = call "ConvStringIntoHex (SubVI).vi"("String In"=w157) -> ("Array Out"=w154:i64[])
        n105 = case shown="\"False\", Default" w169 {
          tunnel: [TRUE TRUE FALSE] -> w168
          frame "False", Default {
          }
          frame "Yes" {
          }
          frame "No" {
          }
        }
        n106 = call "CheckName(SubVI).vi"("Name In"=w167, "Strings And Values[]"=w165) -> ("Name Out"=w166:string)  [unwired: 9 in]
        n107 = Index Array(array=w171, index=0) -> (element=w160:dbl)
        n108 = Index Array(array=w154, index=0) -> (element=w153:i64)
        n109 = Greater?(x=w160, y=w161) -> (0:w162:bool)
        n110 = case shown="True" w162 {
          tunnel: w161 -> [_ w189]
          tunnel: w160 -> [w188 _]
          tunnel: [w188 w189] -> w159
          frame False {
          }
          frame True {
          }
        }
        n111 = property on="Lines" class="Arr (strict)"() -> ("Value"=w164:T3[])  [unwired: 2 in, 2 out]
        n112 = Index Array(array=w164, index=0) -> (element=w184:T3)
        n113 = Bundle By Name(cluster=w184, "Name"=w166, "Array Oy"=w180, "Array Ox"=w178, "Width"=w159, "Color"=w153, "Plot Visible"=w168) -> (w183:T3)
        n114 = Array Size(array=w164) -> (size(s)=w163:i32)
        n115 = Insert Into Array(array=w164, index=w163, new element=w183) -> (w182:T3[])
        n116 = property on="NumPlot" class="DigNum (strict)"("Val(Sgnl)"=w163) -> ()  [unwired: 2 in, 2 out]
        n117 = property on="Lines" class="Arr (strict)"("Val(Sgnl)"=w182) -> ()  [unwired: 2 in, 2 out]
      }
      frame "Change Line" {
        n118 = call "MOKO_Grafic_stm.vi"("StateMachineSteps"=T4[] [{"main stm"=enum."Parse String In", "STM Graph"={"Graph settings"={"Axis X Min"=0.0, "Axis X Name"="", "Axis X Max"=1.0, "Axis Y Min"=0.0, " Axis Y Name"="", "Axis Y Max"=1.0, "Autoscale"=enum."Yes", "Choice Line"=0.0}, "Lines"=[], "Data"=""}}, {"main stm"=enum."Change Data", "STM Graph"={"Graph settings"={"Axis X Min"=0.0, "Axis X Name"="", "Axis X Max"=1.0, "Axis Y Min"=0.0, " Axis Y Name"="", "Axis Y Max"=1.0, "Autoscale"=enum."Yes", "Choice Line"=0.0}, "Lines"=[], "Data"=""}}], "queue in"=w194) -> ()  [unwired: 8 in, 2 out]
      }
      frame "Change Data" {
        w201 = 5.0 ("y")
        n119 = call "MOKO_Grafic_stm.vi"("StateMachineSteps"=T4[] [{"main stm"=enum."Choose ActPlot", "STM Graph"={"Graph settings"={"Axis X Min"=0.0, "Axis X Name"="", "Axis X Max"=1.0, "Axis Y Min"=0.0, " Axis Y Name"="", "Axis Y Max"=1.0, "Autoscale"=enum."Yes", "Choice Line"=0.0}, "Lines"=[], "Data"=""}}, {"main stm"=enum."Set Line Settings", "STM Graph"={"Graph settings"={"Axis X Min"=0.0, "Axis X Name"="", "Axis X Max"=1.0, "Axis Y Min"=0.0, " Axis Y Name"="", "Axis Y Max"=1.0, "Autoscale"=enum."Yes", "Choice Line"=0.0}, "Lines"=[], "Data"=""}}, {"main stm"=enum."Change Combo Box", "STM Graph"={"Graph settings"={"Axis X Min"=0.0, "Axis X Name"="", "Axis X Max"=1.0, "Axis Y Min"=0.0, " Axis Y Name"="", "Axis Y Max"=1.0, "Autoscale"=enum."Yes", "Choice Line"=0.0}, "Lines"=[], "Data"=""}}, {"main stm"=enum."Write Graph", "STM Graph"={"Graph settings"={"Axis X Min"=0.0, "Axis X Name"="", "Axis X Max"=1.0, "Axis Y Min"=0.0, " Axis Y Name"="", "Axis Y Max"=1.0, "Autoscale"=enum."Yes", "Choice Line"=0.0}, "Lines"=[], "Data"=""}}], "queue in"=w237) -> ()  [unwired: 8 in, 2 out]
        n120 = property on="String Array Out" class="Arr (strict)"() -> ("Value"=w219:string[])  [unwired: 2 in, 2 out]
        n121 = Index Array(array=w219, index=0) -> (element=w231:string)
        n122 = Index Array(array=w219, index=1) -> (element=w205:string)
        n123 = Index Array(array=w219, index=2) -> (element=w232:string)
        n124 = Index Array(array=w219, index=3) -> (element=w230:string)
        n125 = Index Array(array=w219, index=4) -> (element=w218:string)
        n126 = Index Array(array=w219, index=5) -> (element=w197:string)
        n127 = Index Array(array=w219, index=6) -> (element=w216:string)
        n128 = call "ConvStringIntoDouble (SubVI).vi"("String In"=w231) -> ("Array Out"=w228:dbl[])
        n129 = call "ConvStringIntoDouble (SubVI).vi"("String In"=w232) -> ("Array Out"=w213:dbl[])
        n130 = call "ConvStringIntoDouble (SubVI).vi"("String In"=w230) -> ("Array Out"=w214:dbl[])
        n131 = call "ConvStringIntoDouble (SubVI).vi"("String In"=w218) -> ("Array Out"=w217:dbl[])
        n132 = call "ConvStringIntoHex (SubVI).vi"("String In"=w197) -> ("Array Out"=w196:i64[])
        n133 = case shown="\"Yes\"" w216 {
          tunnel: [_ TRUE FALSE] -> w215
          frame "False", Default {
          }
          frame "Yes" {
          }
          frame "No" {
          }
        }
        n134 = property on="Lines" class="Arr (strict)"() -> ("Value"=w209:T3[])  [unwired: 2 in, 2 out]
        n135 = Index Array(array=w228, index=0) -> (element=w210:dbl)
        n136 = Index Array(array=w217, index=0) -> (element=w200:dbl)
        n137 = Index Array(array=w209, index=w210) -> (element=w208:T3)
        n138 = property on="Combo Box" class="CmbBox"() -> ("Strings And Values[]"=w204:T8)  [unwired: 2 in, 2 out]
        n139 = Index Array(array=w196, index=0) -> (element=w195:i64)
        n140 = Unbundle By Name(w208) -> ("Name"=w207:string)
        n141 = Greater?(x=w200, y=w201) -> (0:w202:bool)
        n142 = case shown="False" w202 {
          tunnel: w201 -> [_ w239]
          tunnel: w200 -> [w238 _]
          tunnel: [w238 w239] -> w199
          frame False {
          }
          frame True {
          }
        }
        n143 = Equal?(x=w205, y=w207) -> (x = y?=w206:bool)
        n144 = case shown="True" w206 {
          tunnel: w205 -> [w242 w243]
          tunnel: w204 -> [w241 _]
          tunnel: [w240 w243] -> w203
          frame False {
            n145 = call "CheckName(SubVI).vi"("Name In"=w242, "Strings And Values[]"=w241) -> ("Name Out"=w240:string)  [unwired: 9 in]
          }
          frame True {
          }
        }
        n146 = property on="Lines" class="Arr (strict)"() -> ("Value"=w212:T3[])  [unwired: 2 in, 2 out]
        n147 = property on="NumPlot" class="DigNum (strict)"("Val(Sgnl)"=w210) -> ()  [unwired: 2 in, 2 out]
        n148 = Index Array(array=w212, index=0) -> (element=w221:T3)
        n149 = Bundle By Name(cluster=w221, "Name"=w203, "Array Oy"=w213, "Array Ox"=w214, "Width"=w199, "Color"=w195, "Plot Visible"=w215) -> (w222:T3)
        n150 = Replace Array Subset(array=w212, new element=w222, index=w210) -> (w211:T3[])
        n151 = property on="Lines" class="Arr (strict)"("Val(Sgnl)"=w211) -> ()  [unwired: 2 in, 2 out]
      }
      frame "Change Lines" {
        n152 = flat-sequence {
          tunnel: w247 -> [w249]
          tunnel: [w249] -> w246
          tunnel: w246 -> [w250]
          frame #0 {
            n153 = property on="NumPlot" class="DigNum (strict)"("Val(Sgnl)"=0.0 ("Value (Signaling)")) -> ()  [unwired: 2 in, 2 out]
          }
          frame #1 {
            n154 = property on="Lines" class="Arr (strict)"() -> ("Value"=w252:T3[])  [unwired: 2 in, 2 out]
            n155 = for {
              tunnel: w252 -> [_] mode=indexing
              tunnel: w250 -> [w253]
              n156 = call "MOKO_Grafic_stm.vi"("StateMachineSteps"=T4[] [{"main stm"=enum."Choose ActPlot", "STM Graph"={"Graph settings"={"Axis X Min"=0.0, "Axis X Name"="", "Axis X Max"=1.0, "Axis Y Min"=0.0, " Axis Y Name"="", "Axis Y Max"=1.0, "Autoscale"=enum."Yes", "Choice Line"=0.0}, "Lines"=[], "Data"=""}}, {"main stm"=enum."Set Line Settings", "STM Graph"={"Graph settings"={"Axis X Min"=0.0, "Axis X Name"="", "Axis X Max"=1.0, "Axis Y Min"=0.0, " Axis Y Name"="", "Axis Y Max"=1.0, "Autoscale"=enum."Yes", "Choice Line"=0.0}, "Lines"=[], "Data"=""}}, {"main stm"=enum."Increment Smth", "STM Graph"={"Graph settings"={"Axis X Min"=0.0, "Axis X Name"="", "Axis X Max"=1.0, "Axis Y Min"=0.0, " Axis Y Name"="", "Axis Y Max"=1.0, "Autoscale"=enum."Yes", "Choice Line"=0.0}, "Lines"=[], "Data"=""}}], "queue in"=w253) -> ()  [unwired: 8 in, 2 out]
            }
            n157 = call "MOKO_Grafic_stm.vi"("StateMachineSteps"=T4[] [{"main stm"=enum."Set Graph Appearance", "STM Graph"={"Graph settings"={"Axis X Min"=0.0, "Axis X Name"="", "Axis X Max"=1.0, "Axis Y Min"=0.0, " Axis Y Name"="", "Axis Y Max"=1.0, "Autoscale"=enum."Yes", "Choice Line"=0.0}, "Lines"=[], "Data"=""}}], "queue in"=w250) -> ()  [unwired: 8 in, 2 out]
          }
        }
      }
      frame "Change Combo Box" {
        n158 = property on="STM Graph" class="Clust (strict)"() -> ("Value"=w255:T1)  [unwired: 2 in, 2 out]
        n159 = property on="NumPlot" class="DigNum (strict)"() -> ("Value"=w258:dbl)  [unwired: 2 in, 2 out]
        n160 = Unbundle By Name(w255) -> ("Lines"=w261:T3[])
        n161 = Index Array(array=w261, index=w258) -> (element=w260:T3)
        n162 = property on="Combo Box" class="CmbBox"() -> ("Strings And Values[]"=w257:T8)  [unwired: 2 in, 2 out]
        n163 = Unbundle By Name(w260) -> ("Name"=w259:string)
        n164 = call "ChangeComboBox(SubVI).vi"("Name"=w259, "NumPlot"=w258, "Strings and Values In[]"=w257) -> ("Strings and Values Out[]"=w256:cluster{"String":string, "Value":string}[])
        n165 = property on="Combo Box" class="CmbBox"("Strings And Values[]"=w256) -> ()  [unwired: 2 in, 2 out]
      }
      frame "Delete Line" {
        n166 = call "MOKO_Grafic_stm.vi"("StateMachineSteps"=T4[] [{"main stm"=enum."Parse String In", "STM Graph"={"Graph settings"={"Axis X Min"=0.0, "Axis X Name"="", "Axis X Max"=1.0, "Axis Y Min"=0.0, " Axis Y Name"="", "Axis Y Max"=1.0, "Autoscale"=enum."Yes", "Choice Line"=0.0}, "Lines"=[], "Data"=""}}, {"main stm"=enum."Delete Data", "STM Graph"={"Graph settings"={"Axis X Min"=0.0, "Axis X Name"="", "Axis X Max"=1.0, "Axis Y Min"=0.0, " Axis Y Name"="", "Axis Y Max"=1.0, "Autoscale"=enum."Yes", "Choice Line"=0.0}, "Lines"=[], "Data"=""}}, {"main stm"=enum."ReWrite Graph", "STM Graph"={"Graph settings"={"Axis X Min"=0.0, "Axis X Name"="", "Axis X Max"=1.0, "Axis Y Min"=0.0, " Axis Y Name"="", "Axis Y Max"=1.0, "Autoscale"=enum."Yes", "Choice Line"=0.0}, "Lines"=[], "Data"=""}}, {"main stm"=enum."Write Graph", "STM Graph"={"Graph settings"={"Axis X Min"=0.0, "Axis X Name"="", "Axis X Max"=1.0, "Axis Y Min"=0.0, " Axis Y Name"="", "Axis Y Max"=1.0, "Autoscale"=enum."Yes", "Choice Line"=0.0}, "Lines"=[], "Data"=""}}], "queue in"=w263) -> ()  [unwired: 8 in, 2 out]
      }
      frame "Delete Data" {
        n167 = property on="String Array Out" class="Arr (strict)"() -> ("Value"=w270:string[])  [unwired: 2 in, 2 out]
        n168 = Index Array(array=w270, index=0) -> (element=w264:string)
        n169 = case shown="\"False\", Default" w264 {
          tunnel: w264 -> [w278 _]
          tunnel: [w274 _] -> w269
          tunnel: [w273 _] -> w267
          tunnel: [w272 _] -> w266
          frame "False", Default {
            n170 = call "ConvStringIntoDouble (SubVI).vi"("String In"=w278) -> ("Array Out"=w277:dbl[])
            n171 = Sort 1D Array(array=w277) -> (sorted array=w275:dbl[])
            n172 = Array Size(array=w275) -> (size(s)=w276:i32)
            n173 = for {
              shift-right: [w285] -> _
              shift-left: w276 -> [w286]
              tunnel: w275 -> [w287]
              tunnel: w275 -> [_] mode=indexing
              tunnel: [w284] -> w274
              tunnel: [w279] -> w273
              tunnel: [w284] -> w272
              n174 = Decrement(x=w286) -> (x-1=w285:i32)
              n175 = Index Array(array=w287, index=w285) -> (element=w284:dbl)
              n176 = property on="Combo Box" class="CmbBox"() -> ("Strings And Values[]"=w281:T8)  [unwired: 2 in, 2 out]
              n177 = property on="Lines" class="Arr (strict)"() -> ("Value"=w283:T3[])  [unwired: 2 in, 2 out]
              n178 = Delete From Array(array=w283, index=w284) -> (array with subset deleted=w282:T3[])  [unwired: 1 in, 1 out]
              n179 = Increment(x=w284) -> (x+1=w280:dbl)
              n180 = property on="Lines" class="Arr (strict)"("Val(Sgnl)"=w282) -> ()  [unwired: 2 in, 2 out]
              n181 = Delete From Array(array=w281, index=w280) -> (array with subset deleted=w279:T8)  [unwired: 1 in, 1 out]
              n182 = property on="Combo Box" class="CmbBox"("Strings And Values[]"=w279) -> ()  [unwired: 2 in, 2 out]
            }
          }
          frame "All" {
            n183 = property on="Lines" class="Arr (strict)"("Val(Sgnl)"=T3[] [] ("Value (Signaling)")) -> ()  [unwired: 2 in, 2 out]
            n184 = property on="Combo Box" class="CmbBox"("Strings And Values[]"=T8 [{"String"="None", "Value"="-1"}] ("Strings And Values []")) -> ()  [unwired: 2 in, 2 out]
          }
        }
        n185 = property on="NumPlot" class="DigNum (strict)"("Val(Sgnl)"=w266) -> ()  [unwired: 2 in, 2 out]
        n186 = Index Array(array=w267, index=w269) -> (element=w268:cluster{"String":string, "Value":string})
        n187 = Unbundle By Name(w268) -> ("String"=w265:string)
        n188 = property on="Combo Box" class="CmbBox"("Text.Text"=w265) -> ()  [unwired: 2 in, 2 out]
      }
      frame "Set Autoscale" {
        n189 = property on="String Array Out" class="Arr (strict)"() -> ("Value"=w293:string[])  [unwired: 2 in, 2 out]
        n190 = Index Array(array=w293, index=0) -> (element=w291:string)
        n191 = case shown="\"OnlyOx\"" w291 {
          tunnel: [_ enum16{"Yes", "No", "Only Oy", "Only Ox"}."Yes" ("Value") enum16{"Yes", "No", "Only Oy", "Only Ox"}."No" ("Value") enum16{"Yes", "No", "Only Oy", "Only Ox"}."Only Oy" ("Value") enum16{"Yes", "No", "Only Oy", "Only Ox"}."Only Ox" ("Value")] -> w290
          frame "False", Default {
          }
          frame "Yes" {
          }
          frame "No" {
          }
          frame "OnlyOy" {
          }
          frame "OnlyOx" {
          }
        }
        n192 = property on="Autoscale" class="Enum (strict)"("Value"=w290) -> ()  [unwired: 2 in, 2 out]
      }
      frame "Set Graph Appearance" {
        n193 = property on="Graph settings" class="Clust (strict)"() -> ("Value"=w311:T2)  [unwired: 2 in, 2 out]
        n194 = Unbundle By Name(w311) -> ("Axis Y Max"=w305:dbl, "Axis Y Min"=w303:dbl, "Axis X Max"=w301:dbl, "Axis X Min"=w299:dbl, "Autoscale"=w308:enum16{"Yes", "No", "Only Oy", "Only Ox"}, "Axis Y Name"=w310:string, "Axis X Name"=w309:string)
        n195 = property on="XY Graph" class="XYGraph (strict)"("XScale.NameLbl.Text"=w309) -> ()  [unwired: 2 in, 2 out]
        n196 = property on="XY Graph" class="XYGraph (strict)"("YScale.NameLbl.Text"=w310) -> ()  [unwired: 2 in, 2 out]
        n197 = flat-sequence {
          tunnel: w308 -> [w318]
          tunnel: [w312] -> w307
          tunnel: [w313] -> w306
          tunnel: w305 -> [w317]
          tunnel: [w317] -> w304
          tunnel: w303 -> [w316]
          tunnel: [w316] -> w302
          tunnel: w301 -> [w315]
          tunnel: [w315] -> w300
          tunnel: w299 -> [w314]
          tunnel: [w314] -> w298
          tunnel: w307 -> [w332]
          tunnel: w306 -> [w331]
          tunnel: w304 -> [w330]
          tunnel: w302 -> [w329]
          tunnel: w300 -> [w328]
          tunnel: w298 -> [w327]
          frame #0 {
            n198 = case shown="\"Only Ox\"" w318 {
              tunnel: [2 0 0 2] -> w312
              tunnel: [2 0 2 0] -> w313
              frame "Yes", Default {
              }
              frame "No" {
              }
              frame "Only Oy" {
              }
              frame "Only Ox" {
              }
            }
            n199 = property on="XY Graph" class="XYGraph (strict)"("YScale.ScaleFit"=w313) -> ()  [unwired: 2 in, 2 out]
            n200 = property on="XY Graph" class="XYGraph (strict)"("XScale.ScaleFit"=w312) -> ()  [unwired: 2 in, 2 out]
          }
          frame #1 {
            n201 = Equal To 0?(x=w331) -> (x = 0?=w334:bool)
            n202 = Equal To 0?(x=w332) -> (x = 0?=w333:bool)
            n203 = case shown="True" w333 {
              tunnel: w328 -> [_ w336]
              tunnel: w327 -> [_ w335]
              frame False {
              }
              frame True {
                n204 = property on="XY Graph" class="XYGraph (strict)"("XScale.Maximum"=w336) -> ()  [unwired: 2 in, 2 out]
                n205 = property on="XY Graph" class="XYGraph (strict)"("XScale.Minimum"=w335) -> ()  [unwired: 2 in, 2 out]
              }
            }
            n206 = case shown="True" w334 {
              tunnel: w330 -> [_ w338]
              tunnel: w329 -> [_ w337]
              frame False {
              }
              frame True {
                n207 = property on="XY Graph" class="XYGraph (strict)"("YScale.Minimum"=w337) -> ()  [unwired: 2 in, 2 out]
                n208 = property on="XY Graph" class="XYGraph (strict)"("YScale.Maximum"=w338) -> ()  [unwired: 2 in, 2 out]
              }
            }
          }
        }
      }
      frame "Set Line Settings" {
        n209 = property on="STM Graph" class="Clust (strict)"() -> ("Value"=w342:T1)  [unwired: 2 in, 2 out]
        n210 = property on="NumPlot" class="DigNum (strict)"() -> ("Value"=w345:dbl)  [unwired: 2 in, 2 out]
        n211 = Unbundle By Name(w342) -> ("Lines"=w341:T3[])
        n212 = Index Array(array=w341, index=w345) -> (element=w346:T3)
        n213 = Unbundle By Name(w346) -> ("Width"=w343:dbl, "Color"=w339:i64, "Name"=w344:string, "Plot Visible"=w340:bool)
        n214 = property on="XY Graph" class="XYGraph (strict)"("Plot.Line Width"=w343) -> ()  [unwired: 2 in, 2 out]
        n215 = property on="XY Graph" class="XYGraph (strict)"("Plot.Plot Name"=w344) -> ()  [unwired: 2 in, 2 out]
        n216 = property on="XY Graph" class="XYGraph (strict)"("Plot.Visible?"=w340) -> ()  [unwired: 2 in, 2 out]
        n217 = property on="XY Graph" class="XYGraph (strict)"("Plot.Plot Color"=w339) -> ()  [unwired: 2 in, 2 out]
      }
      frame "Get Graph Appearance" {
        n218 = property on="String Array Out" class="Arr (strict)"() -> ("Value"=w349:string[])  [unwired: 2 in, 2 out]
        n219 = Index Array(array=w349, index=0) -> (element=w368:string)
        n220 = Index Array(array=w349, index=1) -> (element=w362:string)
        n221 = Index Array(array=w349, index=2) -> (element=w348:string)
        n222 = call "ConvStringIntoDouble (SubVI).vi"("String In"=w368) -> ("Array Out"=w363:dbl[])
        n223 = call "ConvStringIntoArrayString(SubVI).vi"("String In"=w362) -> ("Array String Out"=w359:string[])
        n224 = case shown="\"False\", Default" w348 {
          tunnel: [w371 enum16{"Yes", "No", "Only Oy", "Only Ox"}."Yes" ("Value") enum16{"Yes", "No", "Only Oy", "Only Ox"}."No" ("Value") enum16{"Yes", "No", "Only Oy", "Only Ox"}."Only Oy" ("Value") enum16{"Yes", "No", "Only Oy", "Only Ox"}."Only Ox" ("Value")] -> w347
          frame "False", Default {
            n225 = property on="Autoscale" class="Enum (strict)"() -> ("Value"=w371:enum16{"Yes", "No", "Only Oy", "Only Ox"})  [unwired: 2 in, 2 out]
          }
          frame "Yes" {
          }
          frame "No" {
          }
          frame "OnlyOy" {
          }
          frame "OnlyOx" {
          }
        }
        n226 = Index Array(array=w363, index=0) -> (element=w357:dbl)
        n227 = Index Array(array=w363, index=1) -> (element=w356:dbl)
        n228 = Index Array(array=w363, index=2) -> (element=w355:dbl)
        n229 = Index Array(array=w363, index=3) -> (element=w354:dbl)
        n230 = Index Array(array=w359, index=0) -> (element=w353:string)
        n231 = Index Array(array=w359, index=1) -> (element=w352:string)
        n232 = property on="Autoscale" class="Enum (strict)"("Value"=w347) -> ()  [unwired: 2 in, 2 out]
        n233 = property on="Graph settings" class="Clust (strict)"() -> ("Value"=w358:T2)  [unwired: 2 in, 2 out]
        n234 = Bundle By Name(cluster=w358, "Axis Y Min"=w357, "Axis Y Max"=w356, "Axis X Min"=w355, "Axis X Max"=w354, "Axis Y Name"=w353, "Axis X Name"=w352, "Autoscale"=w347) -> (w351:T2)
        n235 = property on="Graph settings" class="Clust (strict)"("Val(Sgnl)"=w351) -> ()  [unwired: 2 in, 2 out]
      }
      frame "Get Hide Line" {
        n236 = property on="String Array Out" class="Arr (strict)"() -> ("Value"=w382:string[])  [unwired: 2 in, 2 out]
        n237 = property on="NumPlot" class="DigNum (strict)"("Val(Sgnl)"=0.0 ("Value (Signaling)")) -> ()  [unwired: 2 in, 2 out]
        n238 = Index Array(array=w382, index=0) -> (element=w378:string)
        n239 = property on="Lines" class="Arr (strict)"() -> ("Value"=w376:T3[])  [unwired: 2 in, 2 out]
        n240 = case shown="\"False\", Default" w378 {
          tunnel: w379 -> [w384 w389]
          tunnel: w378 -> [w383 _]
          tunnel: w376 -> [_ w388]
          frame "False", Default {
            n241 = call "ConvStringIntoDouble (SubVI).vi"("String In"=w383) -> ("Array Out"=w385:dbl[])
            "Hide/Show Array" <- w385
            n242 = for {
              tunnel: w385 -> [_] mode=indexing
              tunnel: w384 -> [w386]
              n243 = call "MOKO_Grafic_stm.vi"("StateMachineSteps"=T4[] [{"main stm"=enum."Choose Line", "STM Graph"={"Graph settings"={"Axis X Min"=0.0, "Axis X Name"="", "Axis X Max"=1.0, "Axis Y Min"=0.0, " Axis Y Name"="", "Axis Y Max"=1.0, "Autoscale"=enum."Yes", "Choice Line"=0.0}, "Lines"=[], "Data"=""}}, {"main stm"=enum."Choose ActPlot", "STM Graph"={"Graph settings"={"Axis X Min"=0.0, "Axis X Name"="", "Axis X Max"=1.0, "Axis Y Min"=0.0, " Axis Y Name"="", "Axis Y Max"=1.0, "Autoscale"=enum."Yes", "Choice Line"=0.0}, "Lines"=[], "Data"=""}}, {"main stm"=enum."Hide Data", "STM Graph"={"Graph settings"={"Axis X Min"=0.0, "Axis X Name"="", "Axis X Max"=1.0, "Axis Y Min"=0.0, " Axis Y Name"="", "Axis Y Max"=1.0, "Autoscale"=enum."Yes", "Choice Line"=0.0}, "Lines"=[], "Data"=""}}, {"main stm"=enum."Increment Smth", "STM Graph"={"Graph settings"={"Axis X Min"=0.0, "Axis X Name"="", "Axis X Max"=1.0, "Axis Y Min"=0.0, " Axis Y Name"="", "Axis Y Max"=1.0, "Autoscale"=enum."Yes", "Choice Line"=0.0}, "Lines"=[], "Data"=""}}], "queue in"=w386) -> ()  [unwired: 8 in, 2 out]
            }
          }
          frame "All" {
            n244 = for {
              tunnel: w389 -> [w391]
              tunnel: w388 -> [_] mode=indexing
              n245 = call "MOKO_Grafic_stm.vi"("StateMachineSteps"=T4[] [{"main stm"=enum."Choose ActPlot", "STM Graph"={"Graph settings"={"Axis X Min"=0.0, "Axis X Name"="", "Axis X Max"=1.0, "Axis Y Min"=0.0, " Axis Y Name"="", "Axis Y Max"=1.0, "Autoscale"=enum."Yes", "Choice Line"=0.0}, "Lines"=[], "Data"=""}}, {"main stm"=enum."Increment Smth", "STM Graph"={"Graph settings"={"Axis X Min"=0.0, "Axis X Name"="", "Axis X Max"=1.0, "Axis Y Min"=0.0, " Axis Y Name"="", "Axis Y Max"=1.0, "Autoscale"=enum."Yes", "Choice Line"=0.0}, "Lines"=[], "Data"=""}}, {"main stm"=enum."Hide Data", "STM Graph"={"Graph settings"={"Axis X Min"=0.0, "Axis X Name"="", "Axis X Max"=1.0, "Axis Y Min"=0.0, " Axis Y Name"="", "Axis Y Max"=1.0, "Autoscale"=enum."Yes", "Choice Line"=0.0}, "Lines"=[], "Data"=""}}], "queue in"=w391) -> ()  [unwired: 8 in, 2 out]
            }
          }
        }
        "Counter" <- 0.0 ("Counter")
      }
      frame "Get Show Line" {
        n246 = property on="String Array Out" class="Arr (strict)"() -> ("Value"=w393:string[])  [unwired: 2 in, 2 out]
        n247 = property on="Counter" class="DigNum (strict)"("Val(Sgnl)"=0.0 ("Counter")) -> ()  [unwired: 2 in, 2 out]
        n248 = property on="NumPlot" class="DigNum (strict)"("Val(Sgnl)"=0.0 ("Value (Signaling)")) -> ()  [unwired: 2 in, 2 out]
        n249 = property on="Lines" class="Arr (strict)"() -> ("Value"=w392:T3[])  [unwired: 2 in, 2 out]
        n250 = Index Array(array=w393, index=0) -> (element=w397:string)
        n251 = case shown="\"All\"" w397 {
          tunnel: w396 -> [w403 w412 w429]
          tunnel: w393 -> [w400 w407 _]
          tunnel: w392 -> [_ w406 w428]
          frame "False", Default {
            n252 = Index Array(array=w400, index=1) -> (element=w399:string)
            n253 = call "ConvStringIntoDouble (SubVI).vi"("String In"=w399) -> ("Array Out"=w402:dbl[])
            n254 = property on="Hide/Show Array" class="Arr (strict)"("Val(Sgnl)"=w402) -> ()  [unwired: 2 in, 2 out]
            n255 = for {
              tunnel: w402 -> [_] mode=indexing
              tunnel: w403 -> [w404]
              n256 = call "MOKO_Grafic_stm.vi"("StateMachineSteps"=T4[] [{"main stm"=enum."Choose Line", "STM Graph"={"Graph settings"={"Axis X Min"=0.0, "Axis X Name"="", "Axis X Max"=1.0, "Axis Y Min"=0.0, " Axis Y Name"="", "Axis Y Max"=1.0, "Autoscale"=enum."Yes", "Choice Line"=0.0}, "Lines"=[], "Data"=""}}, {"main stm"=enum."Choose ActPlot", "STM Graph"={"Graph settings"={"Axis X Min"=0.0, "Axis X Name"="", "Axis X Max"=1.0, "Axis Y Min"=0.0, " Axis Y Name"="", "Axis Y Max"=1.0, "Autoscale"=enum."Yes", "Choice Line"=0.0}, "Lines"=[], "Data"=""}}, {"main stm"=enum."Show Data", "STM Graph"={"Graph settings"={"Axis X Min"=0.0, "Axis X Name"="", "Axis X Max"=1.0, "Axis Y Min"=0.0, " Axis Y Name"="", "Axis Y Max"=1.0, "Autoscale"=enum."Yes", "Choice Line"=0.0}, "Lines"=[], "Data"=""}}, {"main stm"=enum."Increment Smth", "STM Graph"={"Graph settings"={"Axis X Min"=0.0, "Axis X Name"="", "Axis X Max"=1.0, "Axis Y Min"=0.0, " Axis Y Name"="", "Axis Y Max"=1.0, "Autoscale"=enum."Yes", "Choice Line"=0.0}, "Lines"=[], "Data"=""}}], "queue in"=w404) -> ()  [unwired: 8 in, 2 out]
            }
          }
          frame "Only" {
            n257 = Index Array(array=w407, index=1) -> (element=w409:string)
            n258 = call "ConvStringIntoDouble (SubVI).vi"("String In"=w409) -> ("Array Out"=w413:dbl[])
            n259 = Sort 1D Array(array=w413) -> (sorted array=w411:dbl[])
            n260 = for {
              tunnel: w412 -> [w420]
              tunnel: w411 -> [w418]
              shift-right: [w417] -> _
              shift-left: 0.0 -> [w416]
              tunnel: w406 -> [_] mode=indexing
              i -> [w414]
              n261 = Index Array(array=w418, index=w416) -> (element=w415:dbl)
              n262 = Equal?(x=w415, y=w414) -> (x = y?=w419:bool)
              n263 = case shown="True" w419 {
                tunnel: w420 -> [w423 w427]
                tunnel: [w421 w425] -> w417
                tunnel: w416 -> [w421 w424]
                frame False {
                  n264 = call "MOKO_Grafic_stm.vi"("StateMachineSteps"=T4[] [{"main stm"=enum."Choose ActPlot", "STM Graph"={"Graph settings"={"Axis X Min"=0.0, "Axis X Name"="", "Axis X Max"=1.0, "Axis Y Min"=0.0, " Axis Y Name"="", "Axis Y Max"=1.0, "Autoscale"=enum."Yes", "Choice Line"=0.0}, "Lines"=[], "Data"=""}}, {"main stm"=enum."Hide Data", "STM Graph"={"Graph settings"={"Axis X Min"=0.0, "Axis X Name"="", "Axis X Max"=1.0, "Axis Y Min"=0.0, " Axis Y Name"="", "Axis Y Max"=1.0, "Autoscale"=enum."Yes", "Choice Line"=0.0}, "Lines"=[], "Data"=""}}, {"main stm"=enum."Increment Smth", "STM Graph"={"Graph settings"={"Axis X Min"=0.0, "Axis X Name"="", "Axis X Max"=1.0, "Axis Y Min"=0.0, " Axis Y Name"="", "Axis Y Max"=1.0, "Autoscale"=enum."Yes", "Choice Line"=0.0}, "Lines"=[], "Data"=""}}], "queue in"=w423) -> ()  [unwired: 8 in, 2 out]
                }
                frame True {
                  n265 = Increment(x=w424) -> (x+1=w425:dbl)
                  n266 = call "MOKO_Grafic_stm.vi"("StateMachineSteps"=T4[] [{"main stm"=enum."Choose ActPlot", "STM Graph"={"Graph settings"={"Axis X Min"=0.0, "Axis X Name"="", "Axis X Max"=1.0, "Axis Y Min"=0.0, " Axis Y Name"="", "Axis Y Max"=1.0, "Autoscale"=enum."Yes", "Choice Line"=0.0}, "Lines"=[], "Data"=""}}, {"main stm"=enum."Show Data", "STM Graph"={"Graph settings"={"Axis X Min"=0.0, "Axis X Name"="", "Axis X Max"=1.0, "Axis Y Min"=0.0, " Axis Y Name"="", "Axis Y Max"=1.0, "Autoscale"=enum."Yes", "Choice Line"=0.0}, "Lines"=[], "Data"=""}}, {"main stm"=enum."Increment Smth", "STM Graph"={"Graph settings"={"Axis X Min"=0.0, "Axis X Name"="", "Axis X Max"=1.0, "Axis Y Min"=0.0, " Axis Y Name"="", "Axis Y Max"=1.0, "Autoscale"=enum."Yes", "Choice Line"=0.0}, "Lines"=[], "Data"=""}}], "queue in"=w427) -> ()  [unwired: 8 in, 2 out]
                }
              }
            }
          }
          frame "All" {
            n267 = for {
              tunnel: w429 -> [w431]
              tunnel: w428 -> [_] mode=indexing
              n268 = call "MOKO_Grafic_stm.vi"("StateMachineSteps"=T4[] [{"main stm"=enum."Choose ActPlot", "STM Graph"={"Graph settings"={"Axis X Min"=0.0, "Axis X Name"="", "Axis X Max"=1.0, "Axis Y Min"=0.0, " Axis Y Name"="", "Axis Y Max"=1.0, "Autoscale"=enum."Yes", "Choice Line"=0.0}, "Lines"=[], "Data"=""}}, {"main stm"=enum."Increment Smth", "STM Graph"={"Graph settings"={"Axis X Min"=0.0, "Axis X Name"="", "Axis X Max"=1.0, "Axis Y Min"=0.0, " Axis Y Name"="", "Axis Y Max"=1.0, "Autoscale"=enum."Yes", "Choice Line"=0.0}, "Lines"=[], "Data"=""}}, {"main stm"=enum."Show Data", "STM Graph"={"Graph settings"={"Axis X Min"=0.0, "Axis X Name"="", "Axis X Max"=1.0, "Axis Y Min"=0.0, " Axis Y Name"="", "Axis Y Max"=1.0, "Autoscale"=enum."Yes", "Choice Line"=0.0}, "Lines"=[], "Data"=""}}], "queue in"=w431) -> ()  [unwired: 8 in, 2 out]
            }
          }
        }
      }
      frame "Hide Line" {
        n269 = call "MOKO_Grafic_stm.vi"("StateMachineSteps"=T4[] [{"main stm"=enum."Parse String In", "STM Graph"={"Graph settings"={"Axis X Min"=0.0, "Axis X Name"="", "Axis X Max"=1.0, "Axis Y Min"=0.0, " Axis Y Name"="", "Axis Y Max"=1.0, "Autoscale"=enum."Yes", "Choice Line"=0.0}, "Lines"=[], "Data"=""}}, {"main stm"=enum."Get Hide Line", "STM Graph"={"Graph settings"={"Axis X Min"=0.0, "Axis X Name"="", "Axis X Max"=1.0, "Axis Y Min"=0.0, " Axis Y Name"="", "Axis Y Max"=1.0, "Autoscale"=enum."Yes", "Choice Line"=0.0}, "Lines"=[], "Data"=""}}], "queue in"=w433) -> ()  [unwired: 8 in, 2 out]
      }
      frame "Hide Data" {
        n270 = property on="XY Graph" class="XYGraph (strict)"("Plot.Visible?"=FALSE ("Plot.Visible")) -> ()  [unwired: 2 in, 2 out]
      }
      frame "Show Line" {
        n271 = call "MOKO_Grafic_stm.vi"("StateMachineSteps"=T4[] [{"main stm"=enum."Parse String In", "STM Graph"={"Graph settings"={"Axis X Min"=0.0, "Axis X Name"="", "Axis X Max"=1.0, "Axis Y Min"=0.0, " Axis Y Name"="", "Axis Y Max"=1.0, "Autoscale"=enum."Yes", "Choice Line"=0.0}, "Lines"=[], "Data"=""}}, {"main stm"=enum."Get Show Line", "STM Graph"={"Graph settings"={"Axis X Min"=0.0, "Axis X Name"="", "Axis X Max"=1.0, "Axis Y Min"=0.0, " Axis Y Name"="", "Axis Y Max"=1.0, "Autoscale"=enum."Yes", "Choice Line"=0.0}, "Lines"=[], "Data"=""}}], "queue in"=w435) -> ()  [unwired: 8 in, 2 out]
      }
      frame "Show Data" {
        n272 = property on="XY Graph" class="XYGraph (strict)"("Plot.Visible?"=TRUE ("Plot.Visible")) -> ()  [unwired: 2 in, 2 out]
      }
      frame "Choose ActPlot" {
        n273 = property on="XY Graph" class="XYGraph (strict)"("Active Plot"="NumPlot") -> ()  [unwired: 2 in, 2 out]
      }
      frame "Choose Line" {
        n274 = property on="Hide/Show Array" class="Arr (strict)"() -> ("Value"=w441:dbl[])  [unwired: 2 in, 2 out]
        n275 = property on="Counter" class="DigNum (strict)"() -> ("Value"=w440:dbl)  [unwired: 2 in, 2 out]
        n276 = Index Array(array=w441, index=w440) -> (element=w439:dbl)
        n277 = property on="NumPlot" class="DigNum (strict)"("Val(Sgnl)"=w439) -> ()  [unwired: 2 in, 2 out]
      }
      frame "Choice Line" {
        n278 = property on="Combo Box" class="CmbBox"() -> ("Strings And Values[]"=w444:T8)  [unwired: 2 in, 2 out]
        n279 = property on="Combo Box" class="CmbBox"() -> ("Text.Text"=w445:string)  [unwired: 2 in, 2 out]
        n280 = while {
          tunnel: w444 -> [w451]
          tunnel: w445 -> [w449]
          tunnel: [w446] -> w443
          i -> [w446]
          stop <- w450 stop-if-true
          n281 = Index Array(array=w451, index=w446) -> (element=w448:cluster{"String":string, "Value":string})
          n282 = Unbundle By Name(w448) -> ("String"=w447:string)
          n283 = Equal?(x=w447, y=w449) -> (x = y?=w450:bool)
        }
        n284 = Decrement(x=w443) -> (x-1=w442:i32)
        n285 = property on="Choice Line" class="DigNum (strict)"("Val(Sgnl)"=w442) -> ()  [unwired: 2 in, 2 out]
      }
      frame "Parse String In" {
        n286 = call "SemiColonParserFromString(SubVI).vi"("String In"="params") -> ("String Array Out"=→"String Array Out":string[])
      }
      frame "Graph Settings" {
        n287 = call "MOKO_Grafic_stm.vi"("StateMachineSteps"=T4[] [{"main stm"=enum."Parse String In", "STM Graph"={"Graph settings"={"Axis X Min"=0.0, "Axis X Name"="", "Axis X Max"=1.0, "Axis Y Min"=0.0, " Axis Y Name"="", "Axis Y Max"=1.0, "Autoscale"=enum."Yes", "Choice Line"=0.0}, "Lines"=[], "Data"=""}}, {"main stm"=enum."Get Graph Appearance", "STM Graph"={"Graph settings"={"Axis X Min"=0.0, "Axis X Name"="", "Axis X Max"=1.0, "Axis Y Min"=0.0, " Axis Y Name"="", "Axis Y Max"=1.0, "Autoscale"=enum."Yes", "Choice Line"=0.0}, "Lines"=[], "Data"=""}}, {"main stm"=enum."Set Graph Appearance", "STM Graph"={"Graph settings"={"Axis X Min"=0.0, "Axis X Name"="", "Axis X Max"=1.0, "Axis Y Min"=0.0, " Axis Y Name"="", "Axis Y Max"=1.0, "Autoscale"=enum."Yes", "Choice Line"=0.0}, "Lines"=[], "Data"=""}}], "queue in"=w455) -> ()  [unwired: 8 in, 2 out]
      }
      frame "Write Graph" {
        n288 = property on="Lines" class="Arr (strict)"() -> ("Value"=w457:T3[])  [unwired: 2 in, 2 out]
        n289 = for {
          tunnel: w457 -> [w461] mode=indexing
          tunnel: [w458] -> w456 mode=indexing
          n290 = Unbundle By Name(w461) -> ("Array Ox"=w460:dbl[], "Array Oy"=w459:dbl[])
          n291 = Bundle("Array Ox"=w460, "Array Oy"=w459) -> (w458:cluster{"Array Ox":dbl[], "Array Oy":dbl[]})  [unwired: 1 in]
        }
        "XY Graph" <- w456
      }
      frame "ReWrite Graph" {
        n292 = property on="Lines" class="Arr (strict)"() -> ("Value"=w462:T3[])  [unwired: 2 in, 2 out]
        n293 = property on="NumPlot" class="DigNum (strict)"() -> ("Value"=w465:dbl)  [unwired: 2 in, 2 out]
        n294 = Array Size(array=w462) -> (size(s)=w466:i32)
        n295 = Subtract(x=w466, y=w465) -> (x-y=w464:dbl)
        n296 = for {
          N: w464 -> [_]
          tunnel: w463 -> [w467]
          n297 = call "MOKO_Grafic_stm.vi"("StateMachineSteps"=T4[] [{"main stm"=enum."Choose ActPlot", "STM Graph"={"Graph settings"={"Axis X Min"=0.0, "Axis X Name"="", "Axis X Max"=1.0, "Axis Y Min"=0.0, " Axis Y Name"="", "Axis Y Max"=1.0, "Autoscale"=enum."Yes", "Choice Line"=0.0}, "Lines"=[], "Data"=""}}, {"main stm"=enum."Set Line Settings", "STM Graph"={"Graph settings"={"Axis X Min"=0.0, "Axis X Name"="", "Axis X Max"=1.0, "Axis Y Min"=0.0, " Axis Y Name"="", "Axis Y Max"=1.0, "Autoscale"=enum."Yes", "Choice Line"=0.0}, "Lines"=[], "Data"=""}}, {"main stm"=enum."Increment Smth", "STM Graph"={"Graph settings"={"Axis X Min"=0.0, "Axis X Name"="", "Axis X Max"=1.0, "Axis Y Min"=0.0, " Axis Y Name"="", "Axis Y Max"=1.0, "Autoscale"=enum."Yes", "Choice Line"=0.0}, "Lines"=[], "Data"=""}}], "queue in"=w467) -> ()  [unwired: 8 in, 2 out]
        }
      }
      frame "Clear Graph" {
        n298 = call "MOKO_Grafic_stm.vi"("StateMachineSteps"=T4[] [{"main stm"=enum."init", "STM Graph"={"Graph settings"={"Axis X Min"=0.0, "Axis X Name"="", "Axis X Max"=1.0, "Axis Y Min"=0.0, " Axis Y Name"="", "Axis Y Max"=1.0, "Autoscale"=enum."Yes", "Choice Line"=0.0}, "Lines"=[], "Data"=""}}], "queue in"=w469) -> ()  [unwired: 8 in, 2 out]
        n299 = disable-structure shown="Disabled" {
          frame Disabled {
            n300 = invoke on="XY Graph" class="XYGraph (strict)" method="Reinit To Default"() -> ()  [unwired: 3 in, 3 out]
          }
          frame Enabled {
          }
        }
      }
      frame "Send Data" {
        n301 = property on="STM Graph" class="Clust (strict)"() -> ("Value"=w474:T1)  [unwired: 2 in, 2 out]
        n302 = Bundle By Name(cluster=T9 {"main stm"=enum."Receive Data", "STM Graph"={"Graph settings"={"Axis X Min"=0.0, "Axis X Name"="", "Axis X Max"=0.0, "Axis Y Min"=0.0, " Axis Y Name"="", "Axis Y Max"=1.0, "Autoscale"=enum."Yes", "Choice Line"=1.0}, "Lines"=[], "Data"=""}} ("MOKO_SE_STM"), "STM Graph"=w474) -> (w473:T9)
        n303 = vi-ref "Graph_Settings.vi"() -> (w471:refnum<vi>)
        n304 = call "OpenAndSendDataToSubVi(SubVI).vi"("reference"=w471, "Control Name"="Graph_Setting", "element"=w473) -> ()  [unwired: 8 in]
      }
      frame "Receive Data" {
        n305 = flat-sequence {
          tunnel: w478 -> [w485]
          tunnel: w477 -> [w484]
          tunnel: [w484] -> w476
          tunnel: w476 -> [w490]
          frame #0 {
            n306 = Unbundle By Name(w485) -> ("Lines"=w486:T3[])
            n307 = property on="STM Graph" class="Clust (strict)"("Val(Sgnl)"=w485) -> ()  [unwired: 2 in, 2 out]
            n308 = for {
              tunnel: w486 -> [w489] mode=indexing
              tunnel: [w487] -> w483 mode=indexing
              n309 = Unbundle By Name(w489) -> ("Name"=w488:string)
              n310 = Bundle("Name"=w488, "Name"=w488) -> (w487:cluster{"Name":string, "Name":string})  [unwired: 1 in]
            }
            n311 = property on="Combo Box" class="CmbBox"() -> ("Value"=w479:string)  [unwired: 2 in, 2 out]
            n312 = Insert Into Array(array=w483, index=0, new element=cluster{"Name":string, "Name":string} {"Name"="None", "Name"="None"} ("new element/subarray")) -> (w480:cluster{"Name":string, "Name":string}[])
            n313 = property on="Combo Box" class="CmbBox"("Val(Sgnl)"=w479) -> ()  [unwired: 2 in, 2 out]
            n314 = property on="Combo Box" class="CmbBox"("Strings And Values[]"=w480) -> ()  [unwired: 2 in, 2 out]
          }
          frame #1 {
            n315 = call "MOKO_Grafic_stm.vi"("StateMachineSteps"=T4[] [{"main stm"=enum."Change Lines", "STM Graph"={"Graph settings"={"Axis X Min"=0.0, "Axis X Name"="", "Axis X Max"=1.0, "Axis Y Min"=0.0, " Axis Y Name"="", "Axis Y Max"=1.0, "Autoscale"=enum."Yes", "Choice Line"=0.0}, "Lines"=[], "Data"=""}}], "queue in"=w490) -> ()  [unwired: 8 in, 2 out]
          }
        }
      }
      frame "Increment Smth" {
        n316 = property on="Counter" class="DigNum (strict)"() -> ("Value"=w493:dbl)  [unwired: 2 in, 2 out]
        n317 = property on="NumPlot" class="DigNum (strict)"() -> ("Value"=w495:dbl)  [unwired: 2 in, 2 out]
        n318 = Increment(x=w495) -> (x+1=w494:dbl)
        n319 = Increment(x=w493) -> (x+1=w492:dbl)
        n320 = property on="NumPlot" class="DigNum (strict)"("Val(Sgnl)"=w494) -> ()  [unwired: 2 in, 2 out]
        n321 = property on="Counter" class="DigNum (strict)"("Val(Sgnl)"=w492) -> ()  [unwired: 2 in, 2 out]
      }
      frame "Autoscale" {
        n322 = call "MOKO_Grafic_stm.vi"("StateMachineSteps"=T4[] [{"main stm"=enum."Parse String In", "STM Graph"={"Graph settings"={"Axis X Min"=0.0, "Axis X Name"="", "Axis X Max"=1.0, "Axis Y Min"=0.0, " Axis Y Name"="", "Axis Y Max"=1.0, "Autoscale"=enum."Yes", "Choice Line"=0.0}, "Lines"=[], "Data"=""}}, {"main stm"=enum."Set Autoscale", "STM Graph"={"Graph settings"={"Axis X Min"=0.0, "Axis X Name"="", "Axis X Max"=1.0, "Axis Y Min"=0.0, " Axis Y Name"="", "Axis Y Max"=1.0, "Autoscale"=enum."Yes", "Choice Line"=0.0}, "Lines"=[], "Data"=""}}, {"main stm"=enum."Set Graph Appearance", "STM Graph"={"Graph settings"={"Axis X Min"=0.0, "Axis X Name"="", "Axis X Max"=1.0, "Axis Y Min"=0.0, " Axis Y Name"="", "Axis Y Max"=1.0, "Autoscale"=enum."Yes", "Choice Line"=0.0}, "Lines"=[], "Data"=""}}], "queue in"=w497) -> ()  [unwired: 8 in, 2 out]
      }
      frame "Screenshot" {
        n323 = flat-sequence {
          frame #0 {
            n324 = property on="Screenshot Indicator" class="Bool (strict)"("Val(Sgnl)"=TRUE ("Value (Signaling)")) -> ()  [unwired: 2 in, 2 out]
          }
          frame #1 {
            w503 = TRUE ("Visible Area Only")
            w507 = enum32{".png", ".jpg", ".bmp"}.".png" ("IMG_FORMAT")
            n325 = call <vilib>:"Application Directory.vi"() -> ("Application Directory"=w509:path)
            n326 = invoke class="VI" method="FP.Get Image"("visible area only"=w503, "image depth"=24 ("Image Depth")) -> ("image data"=w501:T11)  [unwired: 4 in, 5 out]
            n327 = Call Chain() -> (call chain=w506:string[])
            n328 = call "create png.vi"("IMG_FORMAT"=w507, "base path"=w509) -> ("path"=w508:path)  [unwired: 8 in, 1 out]
            n329 = Index Array(array=w506) -> (element=w505:string)  [unwired: 1 in]
            n330 = To Variant(anything=w501) -> (Variant=w502:variant)
            n331 = call "take_screenshot.vi"("Visible area only? (f)"=w503, "IMG_FORMAT"=w507, "Image path"=w508, "vi path"=w505) -> ()  [unwired: 3 in, 2 out]
            n332 = Variant To Flattened String(Variant=w502) -> (data string=w500:string)  [unwired: 1 out]
            n333 = call "Util Convert to Base64 Graph.vi"("String"=w500) -> ("Base64 String"=w499:string)  [unwired: 10 in]
            n334 = property on="Base64 String" class="Str"("Val(Sgnl)"=w499) -> ()  [unwired: 2 in, 2 out]
          }
          frame #2 {
            n335 = property on="Screenshot Indicator" class="Bool (strict)"("Val(Sgnl)"=FALSE ("Value (Signaling)")) -> ()  [unwired: 2 in, 2 out]
          }
        }
      }
    }
  }
  n336 = flat-sequence {
    tunnel: w5 -> [_]
    frame #0 {
      n337 = Current VI's Path() -> (path=w513:path)
      n338 = Path To String(path=w513) -> (string=w514:string)
      n339 = To Lower Case(string=w514) -> (all lower case string=w515:string)
      n340 = Match Pattern(string=w515, regular expression="\\.exe") -> (offset past match=w516:i32)  [unwired: 1 in, 3 out]
      n341 = Greater Than 0?(x=w516) -> (x > 0?=w512:bool)
      n342 = case shown="True" w512 {
        frame False {
          n343 = Stop() -> ()  [unwired: 1 in]
        }
        frame True {
          n344 = Quit LabVIEW() -> ()  [unwired: 1 in]
        }
      }
    }
  }
